vi "Demo_Main-User.vi"() -> ()   [LabVIEW 2010]
uses:
  ControlCAN/ControlCAN.llb/DevType.ctl
  ControlCAN/ControlCAN.llb/CAN Channel.ctl
  ControlCAN/ControlCAN.llb/InitFlag.ctl
  ControlCAN/ControlCAN.llb/Mode.ctl
  ControlCAN/ControlCAN.llb/Fliter.ctl
  ControlCAN/ControlCAN.llb/VCI_CAN_OBJ.ctl
  ControlCAN/ControlCAN.llb/VCI_INIT_CONFIG.ctl
  ControlCAN/ControlCAN.llb/Return Val.ctl
  ControlCAN/ControlCAN.lvlib
panel:
  out "版本号":dbl format="%_3f"
  in  "看门狗周期_R":bool
  in  "看门狗周期":u16
  out "看门狗周期_回":u16
  in  "看门狗周期_W":bool
  in  "看门狗_W":bool
  in  "看门狗":string(combo)="开启"
  in  "监测周期_R":bool
  in  "监测周期":u16
  out "监测周期_回":u16
  in  "监测周期_W":bool
  out "ERRO7":bool
  out "ERRO6":bool
  out "ERRO5":bool
  out "ERRO4":bool
  out "ERRO3":bool
  out "高温":bool
  out "高压":bool
  out "低压":bool
  out "warn7":bool
  out "warn6":bool
  out "warn5":bool
  out "warn4":bool
  out "warn3":bool
  out "高温":bool
  out "warn1":bool
  out "warn0":bool
  out "温度":dbl format="%#.6f"
  out "电机转速":dbl(graph)
  out "CAN ID":u8 format="%x"
  out "数组":u8[](array[numeric]) format="%x"
  in  "DATA_SAVE_W":bool
  out "CI_K0_回":u16
  out "BI_K0_回":u16
  in  "CI_K0_R":bool
  in  "BI_K0_R":bool
  in  "CI_K0_W":bool
  in  "BI_K0_W":bool
  in  "C电流零偏":u16
  in  "B电流零偏":u16
  in  "AI_K0_R":bool
  in  "A电流零偏":u16
  out "AI_K0_回":u16
  in  "AI_K0_W":bool
  out "Sin":i32
  out "Cosin":i32
  in  "加速度_R":bool
  in  "加速度":dbl min=0.0 max=8000.0 format="%#.6f"
  out "加速度_回":dbl format="%#.6f"
  in  "加速度_W":bool
  in  "速度环KI_R":bool
  in  "速度环KP_R":bool
  in  "速度环KI":dbl format="%#.6f"
  out "速度环KI_回":dbl format="%#.6f"
  in  "速度环KI_W":bool
  in  "速度环KP":dbl format="%#.6f"
  out "速度环KP_回":dbl format="%#.6f"
  in  "速度环KP_W":bool
  in  "电流环KI_R":bool
  in  "电流环KP_R":bool
  in  "电流环KI":dbl format="%#.6f"
  out "电流环KI_回":dbl format="%#.6f"
  in  "电流环KI_W":bool
  in  "电流环KP":dbl format="%#.6f"
  out "电流环KP_回":dbl format="%#.6f"
  in  "电流环KP_W":bool
  out "C电流":dbl(graph)
  out "B电流":dbl(graph)
  out "A电流":dbl(graph)
  out "sCnt":u32 caption="处理统计"
  out "模式_回":string(combo)="00"
  in  "模式_R":bool
  in  "设定电流_R":bool
  in  "设定位置_R":bool
  in  "设定速度_R":bool
  in  "存储路径":path
  in  "保存":bool
  out "保存_S":bool
  in  "模式_W":bool
  in  "模式":string(combo)="00"
  in  "设定电流":dbl format="%#.6f"
  out "设定电流_回":dbl format="%#.6f"
  in  "设定电流_W":bool
  in  "设定位置":dbl format="%#.6f"
  out "设定位置_回":dbl format="%#.6f"
  in  "设定位置_W":bool
  in  "设定速度":dbl format="%#.1f"
  out "设定速度_回":dbl format="%#.6f"
  in  "设定速度_W":bool
  in  "监测_W":bool
  in  "监测":string(combo)="30"
  out "电机ID_R":u32
  in  "Clear":bool
  out "Ualfa":dbl format="%#.6f"
  out "Ubate":dbl format="%#.6f"
  out "Uq":dbl format="%#.6f"
  out "Ud":dbl format="%#.6f"
  out "PWM1":u16
  out "PWM2":u16
  out "PWM3":u16
  out "sector":u8
  out "Iqnow":dbl
  out "Idnow":dbl
  out "Ialfa":dbl
  out "Ibeta":dbl
  out "A电流":dbl
  out "C电流":dbl
  out "B电流":dbl
  out "供电电压":dbl
  out "机械角度":dbl format="%.2f"
  out "电气角度":dbl
  out "转速":dbl
  out "CAN STD_ID":u32 format="%x"
  in  "电机ID":string(combo)="00"
  in  "电机ID_W":bool
  out "RecvCnt":u32 caption="接收统计"
  out "SendCnt":u32 caption="发送统计"
  in  "Format":u8(ring) items=["标准帧", "扩展帧"]
  in  "Type":u8(ring) items=["数据帧", "远程帧"]
  in  "Data":string="00 01 02 03 04 05 06 07"
  in  "ID":u32=291 format="0x%x"
  in  "Send":bool
  in  "RcvEnable":bool=TRUE
  out "Open":bool
  in  "Fliter":T1=1 items=["接收所有类型"=1, "只接收标准帧"=2, "只接收扩展帧"=3]
  in  "kBaudRate":u8(ring)=12 caption="波特率" items=["5k bps"=1, "10k bps"=2, "20k bps"=3, "40k bps"=4, "50k bps"=5, "80k bps"=6, "100k bps"=7, "125k bps"=8, "200k bps"=9, "250k bps"=10, "400k bps"=11, "500k bps"=12, "666k bps"=13, "800k bps"=14, "1000k bps"=15, "33.33k bps"=16, "66.66k bps"=17, "83.33k bps"=18]
  in  "Mode":T2 caption="工作模式" items=["正常工作", "仅侦听模式", "自测模式（环回）"]
  in  "InitFlag":T3 caption="初始化参数" items=["使用Flash参数", "使用界面设置参数"]
  in  "AccMask":u32=4294967295 caption="接收屏蔽码" format="%08x"
  in  "AccCode":u32 caption="接收过滤码" format="%08x"
  in  "Close":bool
  in  "Open":bool
  in  "Channel":T4 caption="CAN通道" items=["通道1", "通道2"]
  in  "DevType":T5=3 caption="设备类型" items=["USB-CAN"=2, "USB-CAN2"=3]
  # "CAN分析仪(创-芯-科-技)"
  # "CANalyst-II"
  # "发送指令帧包"
  # "CAN\n  ID"
  # "DATA"
  # "DATA"
  # "DATA"
  # "0"
  # "1"
  # "7"
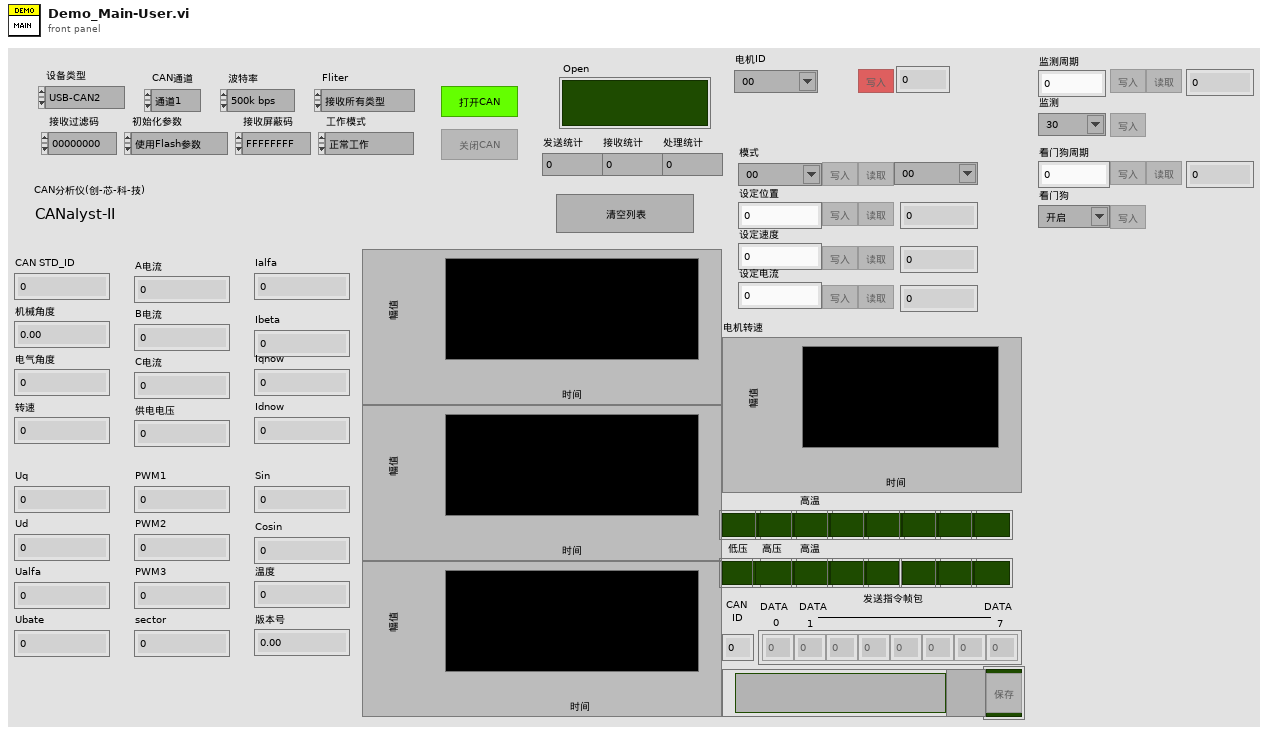
[diagram p1: front panel]
types:
  T1 = typedef "ControlCAN.lvlib/Fliter.ctl" = u8
  T2 = typedef "ControlCAN.lvlib/Mode.ctl" = u8
  T3 = typedef "ControlCAN.lvlib/InitFlag.ctl" = u32
  T4 = typedef "ControlCAN.lvlib/CAN Channel.ctl" = u32
  T5 = typedef "ControlCAN.lvlib/DevType.ctl" = u32
  T6 = typedef "ControlCAN.lvlib/VCI_CAN_OBJ.ctl" = cluster{"ID":u32, "TimeStamp":u32, "TimeFlag":u8, "SendType":u8, "RemoteFlag":u8, "ExternFlag":u8, "DataLen":u8, "Data":u8[], "Reserved":u8[]}
  T7 = cluster{"Type":enum16{"接收", "发送"}, "Channel":T4, "Time":timestamp, "VCI_CAN_OBJ":T6}[]
  T8 = typedef "ControlCAN.lvlib/VCI_INIT_CONFIG.ctl" = cluster{"AccCode":u32, "AccMask":u32, "InitFlag":T3, "Fliter":T1, "Timing0":u8, "Timing1":u8, "Mode":T2}
  T9 = cluster{"DevType":T5, "DevIndex":u32, "CanIndex":T4, "VCI_INIT_CONFIG":T8}
  T10 = typedef "ControlCAN.lvlib/Return Val.ctl" = i32
  T11 = enum16{"open", "replace", "create", "open or create", "replace or create", "replace or create with confirmation"}
  T12 = cluster{"[0]":cluster{"Type":enum16{"接收", "发送"}, "Channel":T4, "Time":timestamp, "VCI_CAN_OBJ":T6}}
  T13 = cluster{"Type":enum16{"接收", "发送"}, "Channel":T4, "Time":timestamp, "VCI_CAN_OBJ":T6}
  T14 = cluster{"Data[0]":u8, "Data[1]":u8, "Data[2]":u8, "Data[3]":u8, "Data[4]":u8, "Data[5]":u8, "Data[6]":u8, "Data[7]":u8}
  T15 = cluster{"Boolean array[0]":bool, "Boolean array[1]":bool, "Boolean array[2]":bool, "Boolean array[3]":bool, "Boolean array[4]":bool, "Boolean array[5]":bool, "Boolean array[6]":bool, "Boolean array[7]":bool}
  T16 = enum32{"invalid app kind", "Development System", "Run Time System", "Student Edition", "Embedded LabVIEW", "Evaluation", "Custom"}
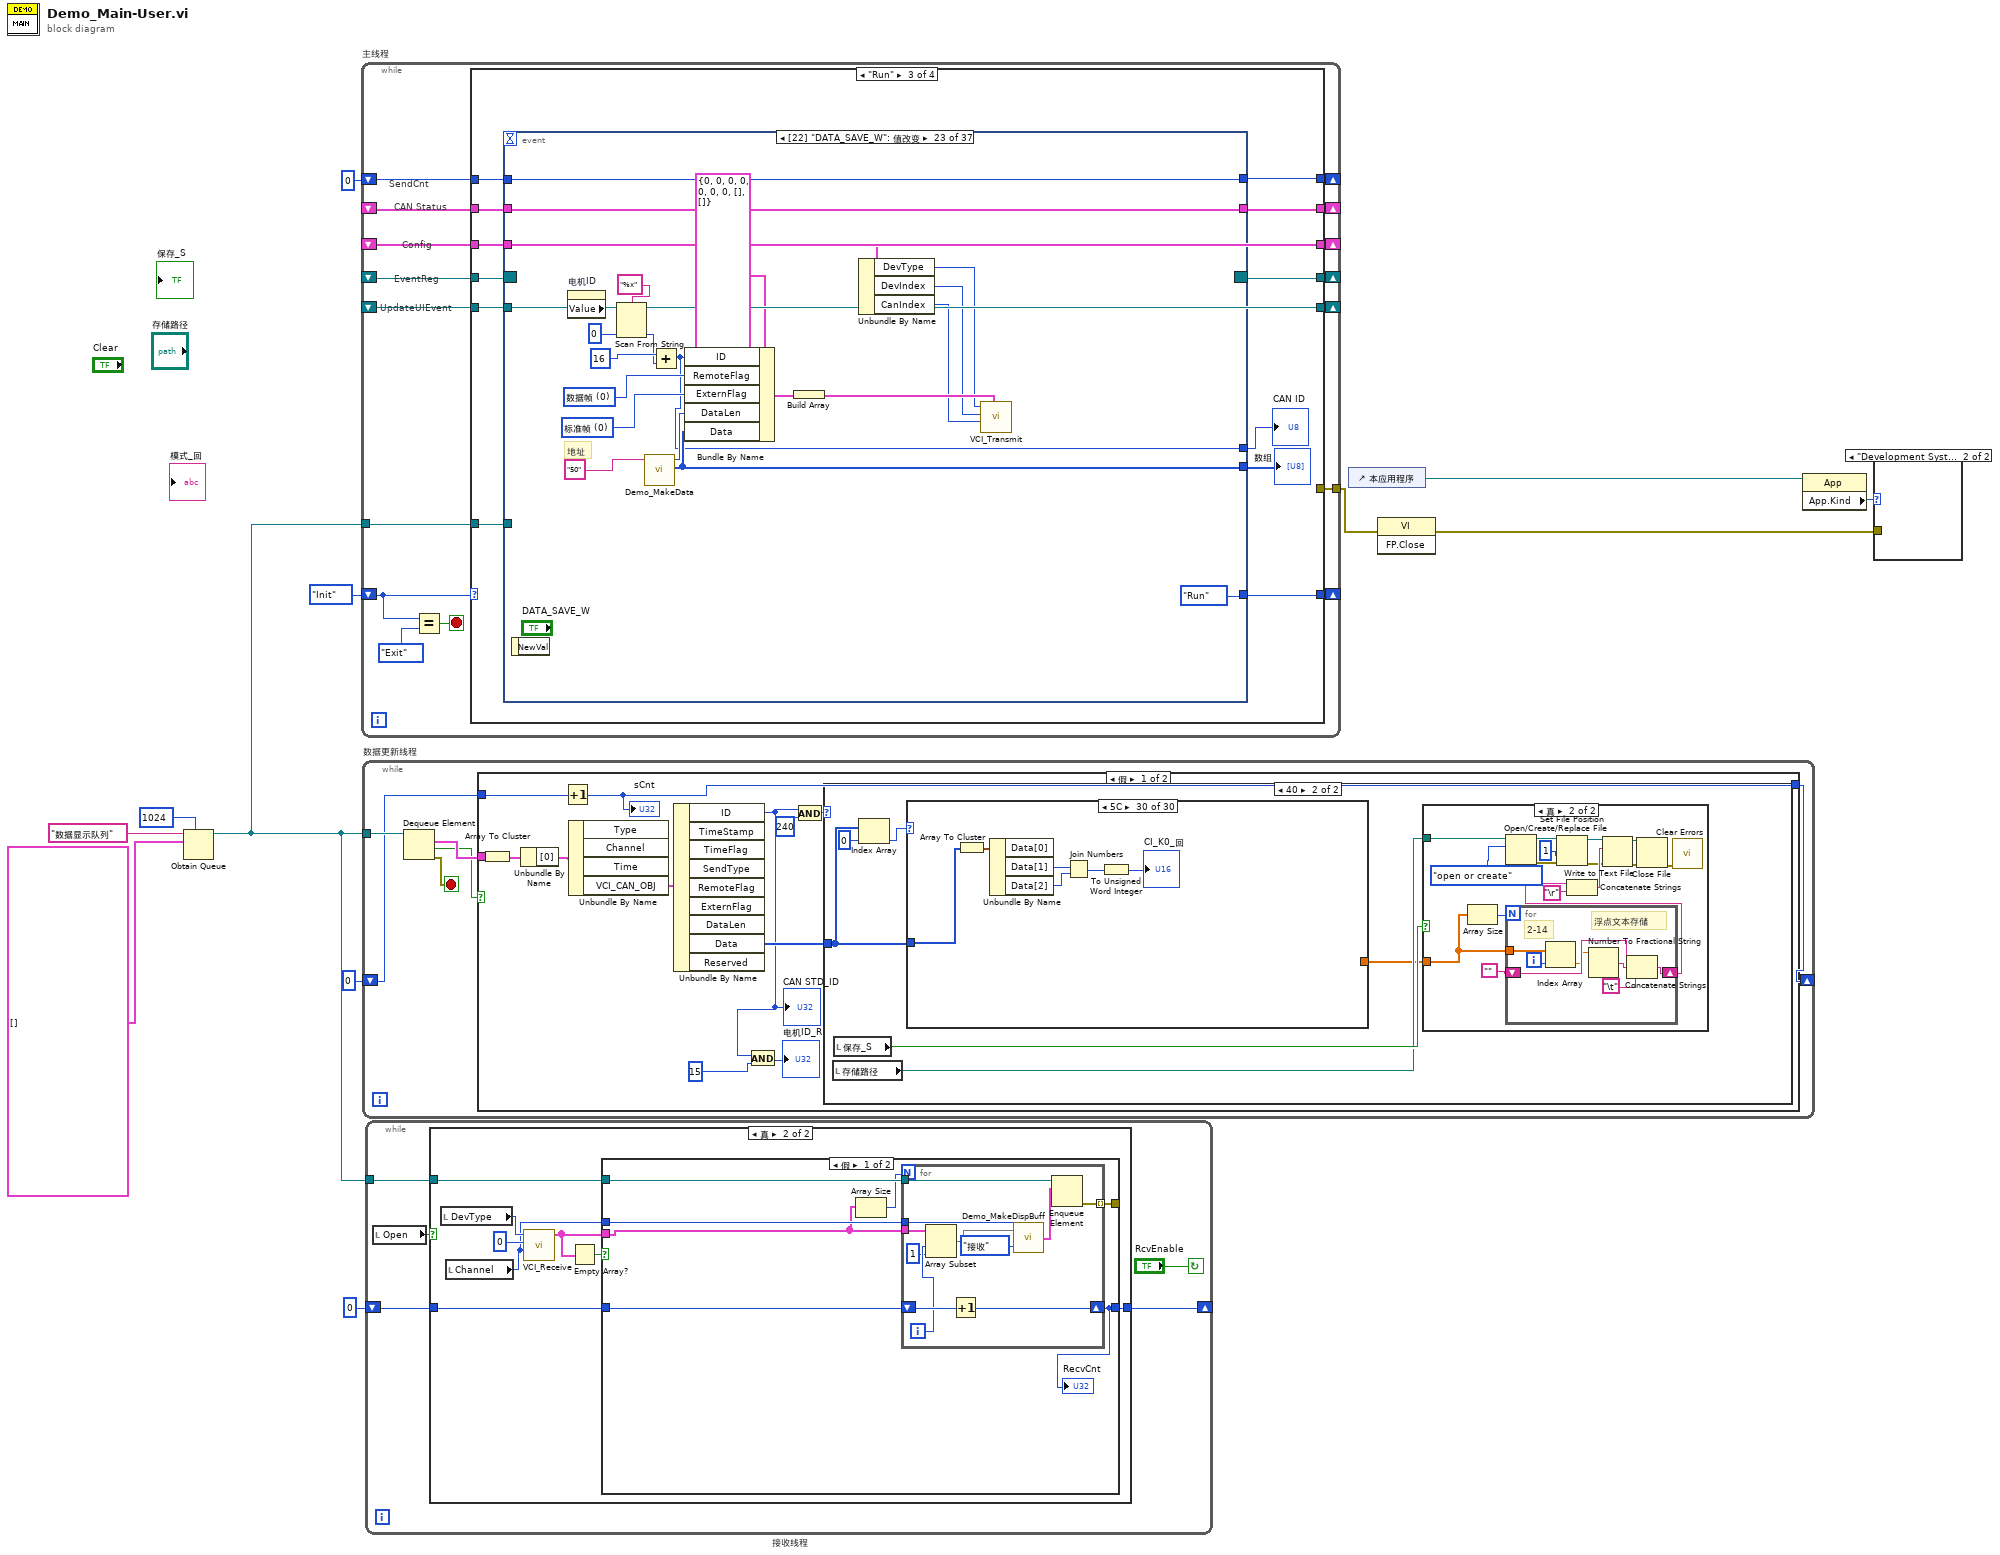
[diagram p0: block diagram]
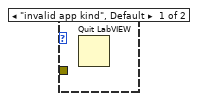
[diagram p2: hidden frame]
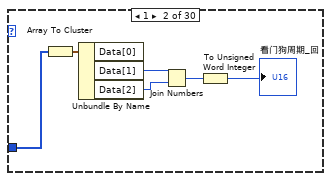
[diagram p6: hidden frame]
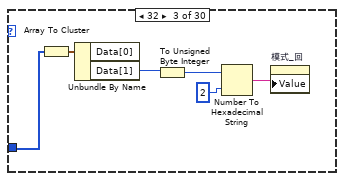
[diagram p7: hidden frame]
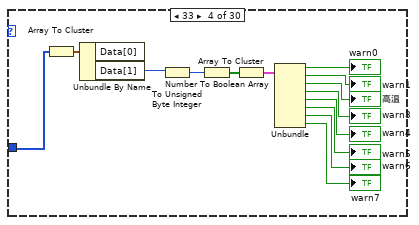
[diagram p8: hidden frame]
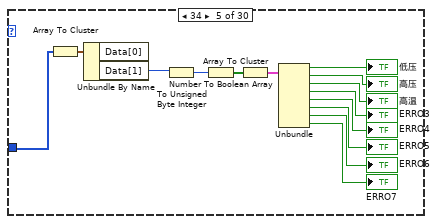
[diagram p9: hidden frame]
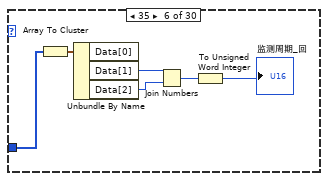
[diagram p10: hidden frame]
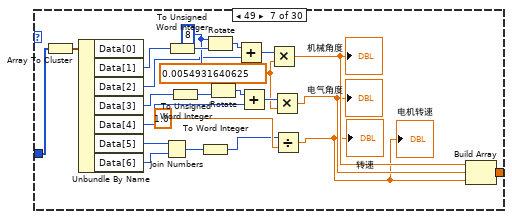
[diagram p11: hidden frame]
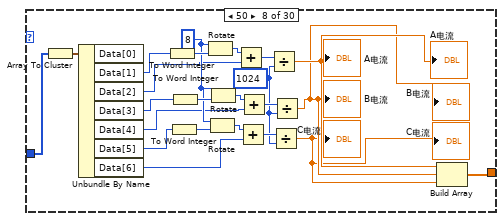
[diagram p12: hidden frame]
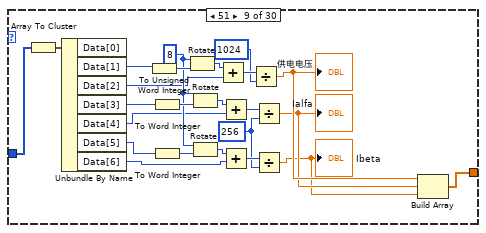
[diagram p13: hidden frame]
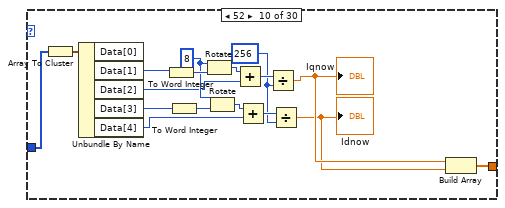
[diagram p14: hidden frame]
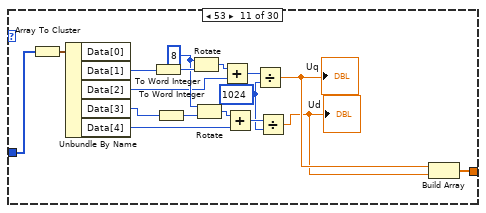
[diagram p15: hidden frame]
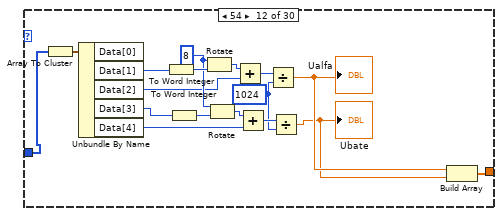
[diagram p16: hidden frame]
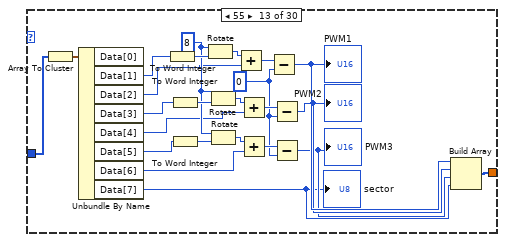
[diagram p17: hidden frame]
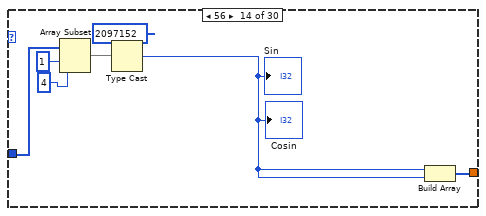
[diagram p18: hidden frame]
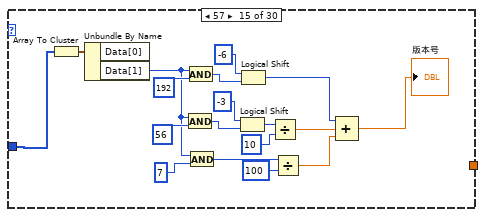
[diagram p19: hidden frame]
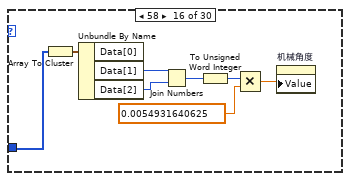
[diagram p20: hidden frame]
diagram:
  n1 = Obtain Queue(max queue size (-1, unlimited)=1024, name (unnamed)="数据显示队列" ("名称（未命名）"), element data type=T7 []) -> (queue out=w9:refnum<queue>)  [unwired: 2 in, 2 out]
  n2 = while "主线程" {
    shift-right: [w24] -> _
    shift-left: enum16{"Init", "Wait", "Run", "Exit"}."Init" -> [w27]
    shift-right: [w25] -> _
    shift-left: _ -> [w26]
    shift-right: [w23] -> _
    shift-left: _ -> [w22]
    tunnel: w9 -> [w21]
    shift-right: [w19] -> _
    shift-left: _ -> [w18]
    shift-right: [w17] -> _
    shift-left: _ -> [w16]
    shift-right: [w14] -> _
    shift-left: u32 0 -> [w15]
    tunnel: [w13] -> w4
    stop <- w28 stop-if-true
    # "CAN Status"
    # "Config"
    # "EventReg"
    # "UpdateUIEvent"
    # "SendCnt"
    n3 = Equal?(x=w27, y=enum16{"Init", "Wait", "Run", "Exit"}."Exit") -> (x = y?=w28:bool)
    n4 = case shown="\"Run\"" w27 {
      tunnel: w26 -> [_ w57 w158 w968]
      tunnel: [w48 w56 w157 w968] -> w25
      tunnel: [enum16{"Init", "Wait", "Run", "Exit"}."Wait" w53 w160 enum16{"Init", "Wait", "Run", "Exit"}."Exit"] -> w24
      tunnel: [w44 w54 w156 w966] -> w23
      tunnel: w22 -> [_ w55 w156 w966]
      tunnel: w21 -> [_ w52 w159 w972]
      tunnel: [w36 w51 w154 w971] -> w19
      tunnel: w18 -> [_ w51 w155 w971]
      tunnel: [w35 w50 w153 w969] -> w17
      tunnel: w16 -> [_ w50 w153 w969]
      tunnel: w15 -> [w33 w49 w152 w964]
      tunnel: [w33 w49 w151 w964] -> w14
      tunnel: [_ _ _ errorcluster {"status"=FALSE, "code"=0, "source"=""} ("error constant")] -> w13
      frame "Init", Default {
        w37 = cluster{"CANOpen":bool} {"CANOpen"=FALSE}  # UpdateUI
        w47 = T9 {"DevType"=2, "DevIndex"=0, "CanIndex"=0, "VCI_INIT_CONFIG"={"AccCode"=0, "AccMask"=0, "InitFlag"=0, "Fliter"=0, "Timing0"=0, "Timing1"=0, "Mode"=0}}  # Config
        w48 = cluster{"Open":bool, "SendCnt":u32} {"Open"=FALSE, "SendCnt"=0}  # CAN Status
        n5 = property class="VI"("Front Panel.Closeable"=TRUE ("前面板窗口:可关闭")) -> ()  [unwired: 2 in, 2 out]
        n6 = invoke class="VI" method="Default Vals.Reinit All"() -> ()  [unwired: 3 in, 3 out]
        n7 = call "Demo_GetT0T1.vi"("kBaudRate"="kBaudRate") -> ("Timing0"=w30:u8, "Timing1"=w29:u8)
        n8 = Bundle By Name(cluster=w47, "DevType"="DevType", "CanIndex"="Channel", "VCI_INIT_CONFIG.AccCode"="AccCode", "VCI_INIT_CONFIG.AccMask"="AccMask", "VCI_INIT_CONFIG.InitFlag"="InitFlag", "VCI_INIT_CONFIG.Fliter"="Fliter", "VCI_INIT_CONFIG.Timing0"=w30, "VCI_INIT_CONFIG.Timing1"=w29, "VCI_INIT_CONFIG.Mode"="Mode") -> (w44:T9)
        n9 = local write "RcvEnable"(TRUE ("RcvEnable")) -> ()
        n10 = Create User Event(user event datatype=w37) -> (user event=w35:refnum<user-event>)  [unwired: 1 in, 1 out]
        n11 = register-events(w35) -> (reference out=w36:refnum<event-registration>)  [unwired: 2 in, 1 out]
      }
      frame "Wait" {
        n12 = event shown="[1] 前面板关闭？" {
          selector: _ -> [_ _ _ _ _ _ _ _ _ _]
          dyn-events: _ -> [_ _ _ _ _ _ _ _ _ _]
          timeout: _ -> [_ _ _ _ _ _ _ _ _ _]
          tunnel: w57 -> [w61 w101 w111 w116 w121 w126 w131 w136 w143 w148]
          tunnel: [w60 w101 w111 w116 w121 w126 w131 w136 w143 w148] -> w56
          tunnel: w55 -> [w71 w100 w110 w115 w120 w125 w130 w135 w142 w147]
          tunnel: [w71 w100 w109 w113 w118 w123 w128 w133 w141 w145] -> w54
          tunnel: [w62 enum16{"Init", "Wait", "Run", "Exit"}."Exit" enum16{"Init", "Wait", "Run", "Exit"}."Wait" enum16{"Init", "Wait", "Run", "Exit"}."Wait" enum16{"Init", "Wait", "Run", "Exit"}."Wait" enum16{"Init", "Wait", "Run", "Exit"}."Wait" enum16{"Init", "Wait", "Run", "Exit"}."Wait" enum16{"Init", "Wait", "Run", "Exit"}."Wait" enum16{"Init", "Wait", "Run", "Exit"}."Wait" enum16{"Init", "Wait", "Run", "Exit"}."Wait"] -> w53
          tunnel: w52 -> [_ _ _ _ _ _ _ _ _ _]
          tunnel: w50 -> [w59 _ _ _ _ _ _ _ _ _]
          event "Open": Value Change {
            w65 = T10 1 items=["OK"=1, "ERROR1"=0, "ERROR2"=-1] ("y")
            # "打开CAN的步骤：\n1.Open\n2.Init\n3.Start"
            n13 = event-data() -> ()  [unwired: 2 out]
            n14 = Unbundle By Name(w71) -> ("DevType"=w70:T5, "DevIndex"=w69:u32)
            n15 = call "VCI_OpenDevice.vi"("DevIndex"=w69, "DevType"=w70) -> ("error out"=w66:errorcluster, "Return Val"=w68:T10)  [unwired: 2 in, 6 out]
            n16 = Equal?(x=w68, y=w65) -> (x = y?=w67:bool)
            n17 = case shown="真" w67 {
              tunnel: w66 -> [_ w86]
              tunnel: w71 -> [_ w85]
              tunnel: w65 -> [_ w77]
              tunnel: [_ w76] -> w58
              frame False {
              }
              frame True {
                n18 = Unbundle By Name(w85) -> ("VCI_INIT_CONFIG"=w84:T8, "DevType"=w80:T5, "DevIndex"=w79:u32, "CanIndex"=w78:T4)
                n19 = call "VCI_InitCAN.vi"("VCI_INIT_CONFIG"=w84, "error in (no error)"=w86, "CANIndex"=w78, "DevIndex"=w79, "DevType"=w80) -> ("error out"=w81:errorcluster, "Return Val"=w83:T10)  [unwired: 5 out]
                n20 = Equal?(x=w77, y=w83) -> (x = y?=w82:bool)
                n21 = case shown="真" w82 {
                  tunnel: w81 -> [_ w97]
                  tunnel: w80 -> [_ w96]
                  tunnel: w79 -> [_ w95]
                  tunnel: w78 -> [_ w94]
                  tunnel: w77 -> [_ w92]
                  tunnel: [_ w88] -> w76
                  frame False {
                  }
                  frame True {
                    n22 = call "VCI_StartCAN.vi"("error in (no error)"=w97, "CANIndex"=w94, "DevIndex"=w95, "DevType"=w96) -> ("error out"=w90:errorcluster, "Return Val"=w93:T10)  [unwired: 6 out]
                    n23 = Unbundle By Name(w90) -> ("status"=w87:bool)
                    n24 = Equal?(x=w92, y=w93) -> (x = y?=w91:bool)
                    n25 = Not(x=w87) -> (.not. x?=w89:bool)
                    n26 = And(x=w91, y=w89) -> (x .and. y?=w88:bool)
                  }
                }
              }
            }
            n27 = case shown="真" w58 {
              tunnel: w59 -> [_ w75]
              tunnel: w58 -> [_ w73]
              frame False {
              }
              frame True {
                n28 = Bundle By Name(cluster=cluster{"CANOpen":bool} {"CANOpen"=FALSE} ("事件数据"), "CANOpen"=w73) -> (w72:cluster{"CANOpen":bool})
                n29 = Generate User Event(user event=w75, event data cluster=w72) -> ()  [unwired: 1 in, 2 out]
              }
            }
            n30 = Select(t=enum16{"Init", "Wait", "Run", "Exit"}."Run", s=w58, f=enum16{"Init", "Wait", "Run", "Exit"}."Wait") -> (s? t:f=w62:enum16{"Init", "Wait", "Run", "Exit"})
            n31 = Bundle By Name(cluster=w61, "Open"=w58) -> (w60:cluster{"Open":bool, "SendCnt":u32})
          }
          event Panel Close? {
            n32 = event-data() -> ()  [unwired: 2 out]
            n33 = event-data("Discard?"=TRUE ("放弃？")) -> ()  [unwired: 1 in, 1 out]
          }
          event Value Change {
            w107 = T5 3 items=["USB-CAN"=2, "USB-CAN2"=3] ("y")
            n34 = event-data() -> ("NewVal"=w108:T5)  [unwired: 1 out]
            n35 = Equal?(x=w108, y=w107) -> (x = y?=w106:bool)
            n36 = Bundle By Name(cluster=w110, "DevType"=w108) -> (w109:T9)
            n37 = Select(t=i32[] [] ("禁用项[]"), s=w106, f=i32[] [1] ("禁用项[]")) -> (s? t:f=w105:i32[])
            n38 = property on="Channel" class="Ring (严格)"("Disabled Items []"=w105) -> ()  [unwired: 2 in, 2 out]
          }
          event Value Change {
            n39 = event-data() -> ("NewVal"=w114:T4)  [unwired: 1 out]
            n40 = Bundle By Name(cluster=w115, "CanIndex"=w114) -> (w113:T9)
          }
          event "AccCode": Value Change {
            n41 = event-data() -> ("NewVal"=w119:u32)  [unwired: 1 out]
            n42 = Bundle By Name(cluster=w120, "VCI_INIT_CONFIG.AccCode"=w119) -> (w118:T9)
          }
          event "AccMask": Value Change {
            n43 = event-data() -> ("NewVal"=w124:u32)  [unwired: 1 out]
            n44 = Bundle By Name(cluster=w125, "VCI_INIT_CONFIG.AccMask"=w124) -> (w123:T9)
          }
          event Value Change {
            n45 = event-data() -> ("NewVal"=w129:T3)  [unwired: 1 out]
            n46 = Bundle By Name(cluster=w130, "VCI_INIT_CONFIG.InitFlag"=w129) -> (w128:T9)
          }
          event Value Change {
            n47 = event-data() -> ("NewVal"=w134:T2)  [unwired: 1 out]
            n48 = Bundle By Name(cluster=w135, "VCI_INIT_CONFIG.Mode"=w134) -> (w133:T9)
          }
          event "kBaudRate": Value Change {
            n49 = event-data() -> ("NewVal"=w139:u8)  [unwired: 1 out]
            n50 = call "Demo_GetT0T1.vi"("kBaudRate"=w139) -> ("Timing0"=w138:u8, "Timing1"=w137:u8)
            n51 = Bundle By Name(cluster=w142, "VCI_INIT_CONFIG.Timing0"=w138, "VCI_INIT_CONFIG.Timing1"=w137) -> (w141:T9)
          }
          event Value Change {
            n52 = event-data() -> ("NewVal"=w146:T1)  [unwired: 1 out]
            n53 = Bundle By Name(cluster=w147, "VCI_INIT_CONFIG.Fliter"=w146) -> (w145:T9)
          }
        }
      }
      frame "Run" {
        n54 = event shown="[22] \"DATA_SAVE_W\": 值改变" {
          selector: w155 -> [_ _ _ _ _ _ _ _ _ _ _ _ _ _ _ _ _ _ _ _ _ _ _ _ _ _ _ _ _ _ _ _ _ _ _ _ _]
          dyn-events: [_ _ _ _ _ _ _ _ _ _ _ _ _ _ _ _ _ _ _ _ _ _ _ _ _ _ _ _ _ _ _ _ _ _ _ _ _] -> w154
          timeout: _ -> [_ _ _ _ _ _ _ _ _ _ _ _ _ _ _ _ _ _ _ _ _ _ _ _ _ _ _ _ _ _ _ _ _ _ _ _ _]
          tunnel: [enum16{"Init", "Wait", "Run", "Exit"}."Run" enum16{"Init", "Wait", "Run", "Exit"}."Run" enum16{"Init", "Wait", "Run", "Exit"}."Run" enum16{"Init", "Wait", "Run", "Exit"}."Run" enum16{"Init", "Wait", "Run", "Exit"}."Run" enum16{"Init", "Wait", "Run", "Exit"}."Run" enum16{"Init", "Wait", "Run", "Exit"}."Run" enum16{"Init", "Wait", "Run", "Exit"}."Run" enum16{"Init", "Wait", "Run", "Exit"}."Run" enum16{"Init", "Wait", "Run", "Exit"}."Run" enum16{"Init", "Wait", "Run", "Exit"}."Run" enum16{"Init", "Wait", "Run", "Exit"}."Run" enum16{"Init", "Wait", "Run", "Exit"}."Run" enum16{"Init", "Wait", "Run", "Exit"}."Run" enum16{"Init", "Wait", "Run", "Exit"}."Run" enum16{"Init", "Wait", "Run", "Exit"}."Run" enum16{"Init", "Wait", "Run", "Exit"}."Run" enum16{"Init", "Wait", "Run", "Exit"}."Run" enum16{"Init", "Wait", "Run", "Exit"}."Run" enum16{"Init", "Wait", "Run", "Exit"}."Run" enum16{"Init", "Wait", "Run", "Exit"}."Run" enum16{"Init", "Wait", "Run", "Exit"}."Run" enum16{"Init", "Wait", "Run", "Exit"}."Run" enum16{"Init", "Wait", "Run", "Exit"}."Run" enum16{"Init", "Wait", "Run", "Exit"}."Run" enum16{"Init", "Wait", "Run", "Exit"}."Run" enum16{"Init", "Wait", "Run", "Exit"}."Run" enum16{"Init", "Wait", "Run", "Exit"}."Run" enum16{"Init", "Wait", "Run", "Exit"}."Run" enum16{"Init", "Wait", "Run", "Exit"}."Run" enum16{"Init", "Wait", "Run", "Exit"}."Run" enum16{"Init", "Wait", "Run", "Exit"}."Run" enum16{"Init", "Wait", "Run", "Exit"}."Run" enum16{"Init", "Wait", "Run", "Exit"}."Run" enum16{"Init", "Wait", "Run", "Exit"}."Run" enum16{"Init", "Wait", "Run", "Exit"}."Run" w957] -> w160
          tunnel: w159 -> [_ _ _ _ _ _ _ _ _ _ _ _ _ _ _ _ _ _ _ _ _ _ _ _ _ _ _ _ _ _ _ _ _ _ _ _ _]
          tunnel: [w162 w179 w196 w220 w241 w262 w281 w302 w318 w356 w377 w403 w429 w455 w481 w507 w533 w559 w585 w609 w633 w657 w678 w699 w720 w741 w762 w783 w804 w825 w846 w867 w888 w909 w937 w943 w962] -> w157
          tunnel: w158 -> [w162 w179 w196 w220 w241 w262 w281 w302 w318 w356 w377 w403 w429 w455 w481 w507 w533 w559 w585 w609 w633 w657 w678 w699 w720 w741 w762 w783 w804 w825 w846 w867 w888 w909 w937 w945 w962]
          tunnel: w156 -> [_ w174 w186 w201 w224 w251 w267 w285 w308 w338 w360 w388 w411 w437 w460 w486 w512 w538 w564 w590 w614 w638 w661 w682 w703 w724 w745 w766 w787 w808 w829 w850 w871 w892 _ w950 _]
          tunnel: w153 -> [_ _ _ _ _ _ _ _ _ _ _ _ _ _ _ _ _ _ _ _ _ _ _ _ _ _ _ _ _ _ _ _ _ _ _ w942 _]
          tunnel: w152 -> [w161 w167 w195 w219 w240 w261 w280 w301 w317 w355 w376 w402 w428 w454 w480 w506 w532 w558 w584 w608 w632 w656 w677 w698 w719 w740 w761 w782 w803 w824 w845 w866 w887 w908 w936 w938 w956]
          tunnel: [w161 w166 w195 w219 w240 w261 w280 w301 w317 w355 w376 w402 w428 w454 w480 w506 w532 w558 w584 w608 w632 w656 w677 w698 w719 w740 w761 w782 w803 w824 w845 w866 w887 w908 w936 w938 w956] -> w151
          tunnel: [_ _ w182 w199 w222 w243 w265 w283 w304 w336 w358 w379 w405 w431 w457 w483 w509 w535 w561 w587 w611 w635 w659 w680 w701 w722 w743 w764 w785 w806 w827 w848 w869 w890 _ _ _] -> w150
          tunnel: [_ _ w181 w200 w223 w242 w266 w284 w307 w335 w357 w378 w404 w430 w456 w482 w508 w534 w560 w586 w610 w634 w658 w679 w700 w721 w742 w763 w784 w805 w826 w847 w868 w889 _ _ _] -> w149
          event Timeout {
            n55 = event-data() -> ()  [unwired: 3 out]
          }
          event "Send": Value Change {
            n56 = event-data() -> ()  [unwired: 2 out]
            n57 = Increment(x=w167) -> (x+1=w166:u32)
            "SendCnt" <- w166
            n58 = call "Demo_MakeData.vi"("DataString"="Data") -> ("Data"=w169:u8[], "DataLen"=w170:u8)  [unwired: 9 out]
            n59 = Bundle By Name(cluster=T6 {"ID"=0, "TimeStamp"=0, "TimeFlag"=0, "SendType"=0, "RemoteFlag"=0, "ExternFlag"=0, "DataLen"=0, "Data"=[], "Reserved"=[]} ("Send"), "ID"="ID", "RemoteFlag"="Type", "ExternFlag"="Format", "DataLen"=w170, "Data"=w169) -> (w164:T6)
            n60 = Build Array(w164) -> (w165:T6[])
            n61 = Unbundle By Name(w174) -> ("DevType"=w173:T5, "DevIndex"=w172:u32, "CanIndex"=w168:T4)
            n62 = call "VCI_Transmit.vi"("Buffer"=w165, "CANIndex"=w168, "DevIndex"=w172, "DevType"=w173) -> ()  [unwired: 1 in, 7 out]
          }
          event "电机ID_W": Value Change {
            w185 = u8 0 items=["数据帧", "遥控帧"]
            w181 = u32 138
            w184 = u8 0 items=["标准帧", "扩展帧"]
            n63 = event-data() -> ()  [unwired: 2 out]
            n64 = call "Demo_MakeData.vi"("DataString"="电机ID") -> ("Data"=w182:u8[], "DataLen"=w190:u8)  [unwired: 9 out]
            n65 = Bundle By Name(cluster=T6 {"ID"=0, "TimeStamp"=0, "TimeFlag"=0, "SendType"=0, "RemoteFlag"=0, "ExternFlag"=0, "DataLen"=0, "Data"=[], "Reserved"=[]} ("Send"), "ID"=w181, "RemoteFlag"=w185, "ExternFlag"=w184, "DataLen"=w190, "Data"=w182) -> (w187:T6)
            n66 = Build Array(w187) -> (w188:T6[])
            n67 = Unbundle By Name(w186) -> ("DevType"=w192:T5, "DevIndex"=w191:u32, "CanIndex"=w189:T4)
            n68 = call "VCI_Transmit.vi"("Buffer"=w188, "CANIndex"=w189, "DevIndex"=w191, "DevType"=w192) -> ()  [unwired: 1 in, 7 out]
          }
          event "监测周期_W": Value Change {
            w213 = u8 0 items=["数据帧", "遥控帧"]
            w214 = u8 0 items=["标准帧", "扩展帧"]
            # "索引地址"
            n69 = event-data() -> ()  [unwired: 2 out]
            n70 = property on="电机ID" class="CmbBox"() -> ("Value"=w205:string)  [unwired: 2 in, 2 out]
            n71 = Scan From String(format string="%x" ("格式字符串"), input string=w205, default 1=u8 0) -> (output 1=w202:u8)  [unwired: 2 in, 3 out]
            n72 = Split Number(x="监测周期") -> (hi(x)=w217:u8, lo(x)=w218:u8)
            n73 = Add(x=u32 16, y=w202) -> (x+y=w200:u32)
            n74 = Build Array(u8 35, w217, w218) -> (w199:u8[])
            n75 = Bundle By Name(cluster=T6 {"ID"=0, "TimeStamp"=0, "TimeFlag"=0, "SendType"=0, "RemoteFlag"=0, "ExternFlag"=0, "DataLen"=0, "Data"=[], "Reserved"=[]} ("Send"), "ID"=w200, "RemoteFlag"=w213, "ExternFlag"=w214, "DataLen"=u8 3, "Data"=w199) -> (w212:T6)
            n76 = Build Array(w212) -> (w211:T6[])
            n77 = Unbundle By Name(w201) -> ("DevType"=w208:T5, "DevIndex"=w209:u32, "CanIndex"=w210:T4)
            n78 = call "VCI_Transmit.vi"("Buffer"=w211, "CANIndex"=w210, "DevIndex"=w209, "DevType"=w208) -> ()  [unwired: 1 in, 7 out]
          }
          event "监测周期_R": Value Change {
            w237 = u8 0 items=["数据帧", "遥控帧"]
            w238 = u8 0 items=["标准帧", "扩展帧"]
            # "地址"
            n79 = event-data() -> ()  [unwired: 2 out]
            n80 = property on="电机ID" class="CmbBox"() -> ("Value"=w228:string)  [unwired: 2 in, 2 out]
            n81 = Scan From String(format string="%x" ("格式字符串"), input string=w228, default 1=u8 0) -> (output 1=w225:u8)  [unwired: 2 in, 3 out]
            n82 = call "Demo_MakeData.vi"("DataString"="23 ") -> ("Data"=w222:u8[], "DataLen"=w233:u8)  [unwired: 9 out]
            n83 = Add(x=u32 48, y=w225) -> (x+y=w223:u32)
            n84 = Bundle By Name(cluster=T6 {"ID"=0, "TimeStamp"=0, "TimeFlag"=0, "SendType"=0, "RemoteFlag"=0, "ExternFlag"=0, "DataLen"=0, "Data"=[], "Reserved"=[]} ("Send"), "ID"=w223, "RemoteFlag"=w237, "ExternFlag"=w238, "DataLen"=w233, "Data"=w222) -> (w236:T6)
            n85 = Build Array(w236) -> (w235:T6[])
            n86 = Unbundle By Name(w224) -> ("DevType"=w231:T5, "DevIndex"=w232:u32, "CanIndex"=w234:T4)
            n87 = call "VCI_Transmit.vi"("Buffer"=w235, "CANIndex"=w234, "DevIndex"=w232, "DevType"=w231) -> ()  [unwired: 1 in, 7 out]
          }
          event "监测_W": Value Change {
            w259 = u8 0 items=["数据帧", "遥控帧"]
            w260 = u8 0 items=["标准帧", "扩展帧"]
            # "地址"
            n88 = event-data() -> ()  [unwired: 2 out]
            n89 = property on="电机ID" class="CmbBox"() -> ("Value"=w248:string)  [unwired: 2 in, 2 out]
            n90 = Scan From String(format string="%x" ("格式字符串"), input string=w248, default 1=u8 0) -> (output 1=w245:u8)  [unwired: 2 in, 3 out]
            n91 = call "Demo_MakeData.vi"("DataString"="监测") -> ("Data"=w243:u8[], "DataLen"=w255:u8)  [unwired: 9 out]
            n92 = Add(x=u32 48, y=w245) -> (x+y=w242:u32)
            n93 = Bundle By Name(cluster=T6 {"ID"=0, "TimeStamp"=0, "TimeFlag"=0, "SendType"=0, "RemoteFlag"=0, "ExternFlag"=0, "DataLen"=0, "Data"=[], "Reserved"=[]} ("Send"), "ID"=w242, "RemoteFlag"=w259, "ExternFlag"=w260, "DataLen"=w255, "Data"=w243) -> (w258:T6)
            n94 = Build Array(w258) -> (w257:T6[])
            n95 = Unbundle By Name(w251) -> ("DevType"=w253:T5, "DevIndex"=w254:u32, "CanIndex"=w256:T4)
            n96 = call "VCI_Transmit.vi"("Buffer"=w257, "CANIndex"=w256, "DevIndex"=w254, "DevType"=w253) -> ()  [unwired: 1 in, 7 out]
          }
          event "看门狗周期_W": Value Change {
            w273 = u8 0 items=["数据帧", "遥控帧"]
            w272 = u8 0 items=["标准帧", "扩展帧"]
            w266 = u32 138
            # "索引地址"
            n97 = event-data() -> ()  [unwired: 2 out]
            n98 = Split Number(x="看门狗周期") -> (hi(x)=w269:u8, lo(x)=w268:u8)
            n99 = Build Array(u8 1, w269, w268) -> (w265:u8[])
            n100 = Bundle By Name(cluster=T6 {"ID"=0, "TimeStamp"=0, "TimeFlag"=0, "SendType"=0, "RemoteFlag"=0, "ExternFlag"=0, "DataLen"=0, "Data"=[], "Reserved"=[]} ("Send"), "ID"=w266, "RemoteFlag"=w273, "ExternFlag"=w272, "DataLen"=u8 3, "Data"=w265) -> (w274:T6)
            n101 = Build Array(w274) -> (w275:T6[])
            n102 = Unbundle By Name(w267) -> ("DevType"=w278:T5, "DevIndex"=w277:u32, "CanIndex"=w276:T4)
            n103 = call "VCI_Transmit.vi"("Buffer"=w275, "CANIndex"=w276, "DevIndex"=w277, "DevType"=w278) -> ()  [unwired: 1 in, 7 out]
          }
          event "看门狗周期_R": Value Change {
            w288 = u8 0 items=["数据帧", "遥控帧"]
            w287 = u8 0 items=["标准帧", "扩展帧"]
            # "地址"
            n104 = event-data() -> ()  [unwired: 2 out]
            n105 = property on="电机ID" class="CmbBox"() -> ("Value"=w297:string)  [unwired: 2 in, 2 out]
            n106 = Scan From String(format string="%x" ("格式字符串"), input string=w297, default 1=u8 0) -> (output 1=w300:u8)  [unwired: 2 in, 3 out]
            n107 = call "Demo_MakeData.vi"("DataString"="01") -> ("Data"=w283:u8[], "DataLen"=w292:u8)  [unwired: 9 out]
            n108 = Add(x=u32 48, y=w300) -> (x+y=w284:u32)
            n109 = Bundle By Name(cluster=T6 {"ID"=0, "TimeStamp"=0, "TimeFlag"=0, "SendType"=0, "RemoteFlag"=0, "ExternFlag"=0, "DataLen"=0, "Data"=[], "Reserved"=[]} ("Send"), "ID"=w284, "RemoteFlag"=w288, "ExternFlag"=w287, "DataLen"=w292, "Data"=w283) -> (w289:T6)
            n110 = Build Array(w289) -> (w290:T6[])
            n111 = Unbundle By Name(w285) -> ("DevType"=w294:T5, "DevIndex"=w293:u32, "CanIndex"=w291:T4)
            n112 = call "VCI_Transmit.vi"("Buffer"=w290, "CANIndex"=w291, "DevIndex"=w293, "DevType"=w294) -> ()  [unwired: 1 in, 7 out]
          }
          event "看门狗_W": Value Change {
            w315 = u8 0 items=["数据帧", "遥控帧"]
            w307 = u32 138
            w316 = u8 0 items=["标准帧", "扩展帧"]
            n113 = event-data() -> ()  [unwired: 2 out]
            n114 = case shown="\"开启\", 默认" "看门狗" {
              tunnel: [w319 w324 w329] -> w304
              frame "开启", Default {
                n115 = Split Number(x=u16 52428) -> (hi(x)=w322:u8, lo(x)=w323:u8)
                n116 = Build Array(u8 2, w322, w323) -> (w319:u8[])
              }
              frame "喂狗" {
                n117 = Split Number(x=u16 43690) -> (hi(x)=w326:u8, lo(x)=w325:u8)
                n118 = Build Array(u8 2, w326, w325) -> (w324:u8[])
              }
              frame "关闭" {
                n119 = Split Number(x=u16 52394) -> (hi(x)=w331:u8, lo(x)=w330:u8)
                n120 = Build Array(u8 2, w331, w330) -> (w329:u8[])
              }
            }
            n121 = Bundle By Name(cluster=T6 {"ID"=0, "TimeStamp"=0, "TimeFlag"=0, "SendType"=0, "RemoteFlag"=0, "ExternFlag"=0, "DataLen"=0, "Data"=[], "Reserved"=[]} ("Send"), "ID"=w307, "RemoteFlag"=w315, "ExternFlag"=w316, "DataLen"=u8 3, "Data"=w304) -> (w314:T6)
            n122 = Build Array(w314) -> (w313:T6[])
            n123 = Unbundle By Name(w308) -> ("DevType"=w310:T5, "DevIndex"=w311:u32, "CanIndex"=w312:T4)
            n124 = call "VCI_Transmit.vi"("Buffer"=w313, "CANIndex"=w312, "DevIndex"=w311, "DevType"=w310) -> ()  [unwired: 1 in, 7 out]
          }
          event "模式_W": Value Change {
            w340 = u8 0 items=["数据帧", "遥控帧"]
            w339 = u8 0 items=["标准帧", "扩展帧"]
            # "地址"
            n125 = event-data() -> ()  [unwired: 2 out]
            n126 = property on="电机ID" class="CmbBox"() -> ("Value"=w349:string)  [unwired: 2 in, 2 out]
            n127 = Concatenate Strings("20 ", "模式") -> (w353:string)
            n128 = Scan From String(format string="%x" ("格式字符串"), input string=w349, default 1=u8 0) -> (output 1=w352:u8)  [unwired: 2 in, 3 out]
            n129 = property on="模式_回" class="CmbBox"("Value"="模式") -> ()  [unwired: 2 in, 2 out]
            n130 = call "Demo_MakeData.vi"("DataString"=w353) -> ("Data"=w336:u8[], "DataLen"=w344:u8)  [unwired: 9 out]
            n131 = Add(x=u32 16, y=w352) -> (x+y=w335:u32)
            n132 = Bundle By Name(cluster=T6 {"ID"=0, "TimeStamp"=0, "TimeFlag"=0, "SendType"=0, "RemoteFlag"=0, "ExternFlag"=0, "DataLen"=0, "Data"=[], "Reserved"=[]} ("Send"), "ID"=w335, "RemoteFlag"=w340, "ExternFlag"=w339, "DataLen"=w344, "Data"=w336) -> (w341:T6)
            n133 = Build Array(w341) -> (w342:T6[])
            n134 = Unbundle By Name(w338) -> ("DevType"=w346:T5, "DevIndex"=w345:u32, "CanIndex"=w343:T4)
            n135 = call "VCI_Transmit.vi"("Buffer"=w342, "CANIndex"=w343, "DevIndex"=w345, "DevType"=w346) -> ()  [unwired: 1 in, 7 out]
          }
          event "模式_R": Value Change {
            w373 = u8 0 items=["数据帧", "遥控帧"]
            w374 = u8 0 items=["标准帧", "扩展帧"]
            # "地址"
            n136 = event-data() -> ()  [unwired: 2 out]
            n137 = property on="电机ID" class="CmbBox"() -> ("Value"=w364:string)  [unwired: 2 in, 2 out]
            n138 = Scan From String(format string="%x" ("格式字符串"), input string=w364, default 1=u8 0) -> (output 1=w361:u8)  [unwired: 2 in, 3 out]
            n139 = call "Demo_MakeData.vi"("DataString"="20 ") -> ("Data"=w358:u8[], "DataLen"=w369:u8)  [unwired: 9 out]
            n140 = Add(x=u32 48, y=w361) -> (x+y=w357:u32)
            n141 = Bundle By Name(cluster=T6 {"ID"=0, "TimeStamp"=0, "TimeFlag"=0, "SendType"=0, "RemoteFlag"=0, "ExternFlag"=0, "DataLen"=0, "Data"=[], "Reserved"=[]} ("Send"), "ID"=w357, "RemoteFlag"=w373, "ExternFlag"=w374, "DataLen"=w369, "Data"=w358) -> (w372:T6)
            n142 = Build Array(w372) -> (w371:T6[])
            n143 = Unbundle By Name(w360) -> ("DevType"=w367:T5, "DevIndex"=w368:u32, "CanIndex"=w370:T4)
            n144 = call "VCI_Transmit.vi"("Buffer"=w371, "CANIndex"=w370, "DevIndex"=w368, "DevType"=w367) -> ()  [unwired: 1 in, 7 out]
          }
          event "设定位置_W": Value Change {
            w390 = u8 0 items=["数据帧", "遥控帧"]
            w389 = u8 0 items=["标准帧", "扩展帧"]
            # "索引地址"
            n145 = event-data() -> ()  [unwired: 2 out]
            n146 = property on="电机ID" class="CmbBox"() -> ("Value"=w398:string)  [unwired: 2 in, 2 out]
            n147 = Multiply ("乘")(x="设定位置", y=u16 256) -> (x*y=w382:i16)
            n148 = Scan From String(format string="%x" ("格式字符串"), input string=w398, default 1=u8 0) -> (output 1=w401:u8)  [unwired: 2 in, 3 out]
            n149 = Split Number(x=w382) -> (hi(x)=w381:u8, lo(x)=w380:u8)
            n150 = Add(x=u32 16, y=w401) -> (x+y=w378:u32)
            n151 = Build Array(u8 64, w381, w380) -> (w379:u8[])
            n152 = Bundle By Name(cluster=T6 {"ID"=0, "TimeStamp"=0, "TimeFlag"=0, "SendType"=0, "RemoteFlag"=0, "ExternFlag"=0, "DataLen"=0, "Data"=[], "Reserved"=[]} ("Send"), "ID"=w378, "RemoteFlag"=w390, "ExternFlag"=w389, "DataLen"=u8 3, "Data"=w379) -> (w391:T6)
            n153 = Build Array(w391) -> (w392:T6[])
            n154 = Unbundle By Name(w388) -> ("DevType"=w395:T5, "DevIndex"=w394:u32, "CanIndex"=w393:T4)
            n155 = call "VCI_Transmit.vi"("Buffer"=w392, "CANIndex"=w393, "DevIndex"=w394, "DevType"=w395) -> ()  [unwired: 1 in, 7 out]
          }
          event "设定速度_W": Value Change {
            w423 = u8 0 items=["数据帧", "遥控帧"]
            w424 = u8 0 items=["标准帧", "扩展帧"]
            # "索引地址"
            n156 = event-data() -> ()  [unwired: 2 out]
            n157 = property on="电机ID" class="CmbBox"() -> ("Value"=w415:string)  [unwired: 2 in, 2 out]
            n158 = Multiply ("乘")(x="设定速度", y=i16 1) -> (x*y=w408:i16)
            n159 = Scan From String(format string="%x" ("格式字符串"), input string=w415, default 1=u8 0) -> (output 1=w412:u8)  [unwired: 2 in, 3 out]
            n160 = Split Number(x=w408) -> (hi(x)=w407:u8, lo(x)=w406:u8)
            n161 = Add(x=u32 16, y=w412) -> (x+y=w404:u32)
            n162 = Build Array(u8 65, w407, w406) -> (w405:u8[])
            n163 = Bundle By Name(cluster=T6 {"ID"=0, "TimeStamp"=0, "TimeFlag"=0, "SendType"=0, "RemoteFlag"=0, "ExternFlag"=0, "DataLen"=0, "Data"=[], "Reserved"=[]} ("Send"), "ID"=w404, "RemoteFlag"=w423, "ExternFlag"=w424, "DataLen"=u8 3, "Data"=w405) -> (w422:T6)
            n164 = Build Array(w422) -> (w421:T6[])
            n165 = Unbundle By Name(w411) -> ("DevType"=w418:T5, "DevIndex"=w419:u32, "CanIndex"=w420:T4)
            n166 = call "VCI_Transmit.vi"("Buffer"=w421, "CANIndex"=w420, "DevIndex"=w419, "DevType"=w418) -> ()  [unwired: 1 in, 7 out]
          }
          event "设定电流_W": Value Change {
            w442 = u8 0 items=["数据帧", "遥控帧"]
            w441 = u8 0 items=["标准帧", "扩展帧"]
            # "索引地址"
            n167 = event-data() -> ()  [unwired: 2 out]
            n168 = property on="电机ID" class="CmbBox"() -> ("Value"=w450:string)  [unwired: 2 in, 2 out]
            n169 = Multiply ("乘")(x="设定电流", y=i16 256) -> (x*y=w434:i16)
            n170 = Scan From String(format string="%x" ("格式字符串"), input string=w450, default 1=u8 0) -> (output 1=w453:u8)  [unwired: 2 in, 3 out]
            n171 = Split Number(x=w434) -> (hi(x)=w433:u8, lo(x)=w432:u8)
            n172 = Add(x=u32 16, y=w453) -> (x+y=w430:u32)
            n173 = Build Array(u8 66, w433, w432) -> (w431:u8[])
            n174 = Bundle By Name(cluster=T6 {"ID"=0, "TimeStamp"=0, "TimeFlag"=0, "SendType"=0, "RemoteFlag"=0, "ExternFlag"=0, "DataLen"=0, "Data"=[], "Reserved"=[]} ("Send"), "ID"=w430, "RemoteFlag"=w442, "ExternFlag"=w441, "DataLen"=u8 3, "Data"=w431) -> (w443:T6)
            n175 = Build Array(w443) -> (w444:T6[])
            n176 = Unbundle By Name(w437) -> ("DevType"=w447:T5, "DevIndex"=w446:u32, "CanIndex"=w445:T4)
            n177 = call "VCI_Transmit.vi"("Buffer"=w444, "CANIndex"=w445, "DevIndex"=w446, "DevType"=w447) -> ()  [unwired: 1 in, 7 out]
          }
          event "电流环KP_W": Value Change {
            w472 = u8 0 items=["数据帧", "遥控帧"]
            w473 = u8 0 items=["标准帧", "扩展帧"]
            # "索引地址"
            n178 = event-data() -> ()  [unwired: 2 out]
            n179 = property on="电机ID" class="CmbBox"() -> ("Value"=w464:string)  [unwired: 2 in, 2 out]
            n180 = Multiply ("乘")(x="电流环KP", y=u16 256) -> (x*y=w477:u16)
            n181 = Scan From String(format string="%x" ("格式字符串"), input string=w464, default 1=u8 0) -> (output 1=w461:u8)  [unwired: 2 in, 3 out]
            n182 = Split Number(x=w477) -> (hi(x)=w478:u8, lo(x)=w479:u8)
            n183 = Add(x=u32 16, y=w461) -> (x+y=w456:u32)
            n184 = Build Array(u8 81, w478, w479) -> (w457:u8[])
            n185 = Bundle By Name(cluster=T6 {"ID"=0, "TimeStamp"=0, "TimeFlag"=0, "SendType"=0, "RemoteFlag"=0, "ExternFlag"=0, "DataLen"=0, "Data"=[], "Reserved"=[]} ("Send"), "ID"=w456, "RemoteFlag"=w472, "ExternFlag"=w473, "DataLen"=u8 3, "Data"=w457) -> (w471:T6)
            n186 = Build Array(w471) -> (w470:T6[])
            n187 = Unbundle By Name(w460) -> ("DevType"=w467:T5, "DevIndex"=w468:u32, "CanIndex"=w469:T4)
            n188 = call "VCI_Transmit.vi"("Buffer"=w470, "CANIndex"=w469, "DevIndex"=w468, "DevType"=w467) -> ()  [unwired: 1 in, 7 out]
          }
          event "电流环KI_W": Value Change {
            w494 = u8 0 items=["数据帧", "遥控帧"]
            w493 = u8 0 items=["标准帧", "扩展帧"]
            # "索引地址"
            n189 = event-data() -> ()  [unwired: 2 out]
            n190 = property on="电机ID" class="CmbBox"() -> ("Value"=w502:string)  [unwired: 2 in, 2 out]
            n191 = Multiply ("乘")(x="电流环KI", y=u16 256) -> (x*y=w489:u16)
            n192 = Scan From String(format string="%x" ("格式字符串"), input string=w502, default 1=u8 0) -> (output 1=w505:u8)  [unwired: 2 in, 3 out]
            n193 = Split Number(x=w489) -> (hi(x)=w488:u8, lo(x)=w487:u8)
            n194 = Add(x=u32 16, y=w505) -> (x+y=w482:u32)
            n195 = Build Array(u8 82, w488, w487) -> (w483:u8[])
            n196 = Bundle By Name(cluster=T6 {"ID"=0, "TimeStamp"=0, "TimeFlag"=0, "SendType"=0, "RemoteFlag"=0, "ExternFlag"=0, "DataLen"=0, "Data"=[], "Reserved"=[]} ("Send"), "ID"=w482, "RemoteFlag"=w494, "ExternFlag"=w493, "DataLen"=u8 3, "Data"=w483) -> (w495:T6)
            n197 = Build Array(w495) -> (w496:T6[])
            n198 = Unbundle By Name(w486) -> ("DevType"=w499:T5, "DevIndex"=w498:u32, "CanIndex"=w497:T4)
            n199 = call "VCI_Transmit.vi"("Buffer"=w496, "CANIndex"=w497, "DevIndex"=w498, "DevType"=w499) -> ()  [unwired: 1 in, 7 out]
          }
          event "速度环KP_W": Value Change {
            w520 = u8 0 items=["数据帧", "遥控帧"]
            w519 = u8 0 items=["标准帧", "扩展帧"]
            # "索引地址"
            n200 = event-data() -> ()  [unwired: 2 out]
            n201 = property on="电机ID" class="CmbBox"() -> ("Value"=w528:string)  [unwired: 2 in, 2 out]
            n202 = Multiply ("乘")(x="速度环KP", y=u16 256) -> (x*y=w515:u16)
            n203 = Scan From String(format string="%x" ("格式字符串"), input string=w528, default 1=u8 0) -> (output 1=w531:u8)  [unwired: 2 in, 3 out]
            n204 = Split Number(x=w515) -> (hi(x)=w514:u8, lo(x)=w513:u8)
            n205 = Add(x=u32 16, y=w531) -> (x+y=w508:u32)
            n206 = Build Array(u8 83, w514, w513) -> (w509:u8[])
            n207 = Bundle By Name(cluster=T6 {"ID"=0, "TimeStamp"=0, "TimeFlag"=0, "SendType"=0, "RemoteFlag"=0, "ExternFlag"=0, "DataLen"=0, "Data"=[], "Reserved"=[]} ("Send"), "ID"=w508, "RemoteFlag"=w520, "ExternFlag"=w519, "DataLen"=u8 3, "Data"=w509) -> (w521:T6)
            n208 = Build Array(w521) -> (w522:T6[])
            n209 = Unbundle By Name(w512) -> ("DevType"=w525:T5, "DevIndex"=w524:u32, "CanIndex"=w523:T4)
            n210 = call "VCI_Transmit.vi"("Buffer"=w522, "CANIndex"=w523, "DevIndex"=w524, "DevType"=w525) -> ()  [unwired: 1 in, 7 out]
          }
          event "速度环KI_W": Value Change {
            w550 = u8 0 items=["数据帧", "遥控帧"]
            w551 = u8 0 items=["标准帧", "扩展帧"]
            # "索引地址"
            n211 = event-data() -> ()  [unwired: 2 out]
            n212 = property on="电机ID" class="CmbBox"() -> ("Value"=w542:string)  [unwired: 2 in, 2 out]
            n213 = Multiply ("乘")(x="速度环KI", y=u16 256) -> (x*y=w555:u16)
            n214 = Scan From String(format string="%x" ("格式字符串"), input string=w542, default 1=u8 0) -> (output 1=w539:u8)  [unwired: 2 in, 3 out]
            n215 = Split Number(x=w555) -> (hi(x)=w556:u8, lo(x)=w557:u8)
            n216 = Add(x=u32 16, y=w539) -> (x+y=w534:u32)
            n217 = Build Array(u8 84, w556, w557) -> (w535:u8[])
            n218 = Bundle By Name(cluster=T6 {"ID"=0, "TimeStamp"=0, "TimeFlag"=0, "SendType"=0, "RemoteFlag"=0, "ExternFlag"=0, "DataLen"=0, "Data"=[], "Reserved"=[]} ("Send"), "ID"=w534, "RemoteFlag"=w550, "ExternFlag"=w551, "DataLen"=u8 3, "Data"=w535) -> (w549:T6)
            n219 = Build Array(w549) -> (w548:T6[])
            n220 = Unbundle By Name(w538) -> ("DevType"=w545:T5, "DevIndex"=w546:u32, "CanIndex"=w547:T4)
            n221 = call "VCI_Transmit.vi"("Buffer"=w548, "CANIndex"=w547, "DevIndex"=w546, "DevType"=w545) -> ()  [unwired: 1 in, 7 out]
          }
          event "加速度_W": Value Change {
            w572 = u8 0 items=["数据帧", "遥控帧"]
            w571 = u8 0 items=["标准帧", "扩展帧"]
            # "索引地址"
            n222 = event-data() -> ()  [unwired: 2 out]
            n223 = property on="电机ID" class="CmbBox"() -> ("Value"=w580:string)  [unwired: 2 in, 2 out]
            n224 = Multiply ("乘")(x="加速度", y=u16 8) -> (x*y=w567:u16)
            n225 = Scan From String(format string="%x" ("格式字符串"), input string=w580, default 1=u8 0) -> (output 1=w583:u8)  [unwired: 2 in, 3 out]
            n226 = Split Number(x=w567) -> (hi(x)=w566:u8, lo(x)=w565:u8)
            n227 = Add(x=u32 16, y=w583) -> (x+y=w560:u32)
            n228 = Build Array(u8 85, w566, w565) -> (w561:u8[])
            n229 = Bundle By Name(cluster=T6 {"ID"=0, "TimeStamp"=0, "TimeFlag"=0, "SendType"=0, "RemoteFlag"=0, "ExternFlag"=0, "DataLen"=0, "Data"=[], "Reserved"=[]} ("Send"), "ID"=w560, "RemoteFlag"=w572, "ExternFlag"=w571, "DataLen"=u8 3, "Data"=w561) -> (w573:T6)
            n230 = Build Array(w573) -> (w574:T6[])
            n231 = Unbundle By Name(w564) -> ("DevType"=w577:T5, "DevIndex"=w576:u32, "CanIndex"=w575:T4)
            n232 = call "VCI_Transmit.vi"("Buffer"=w574, "CANIndex"=w575, "DevIndex"=w576, "DevType"=w577) -> ()  [unwired: 1 in, 7 out]
          }
          event "AI_K0_W": Value Change {
            w596 = u8 0 items=["数据帧", "遥控帧"]
            w595 = u8 0 items=["标准帧", "扩展帧"]
            # "索引地址"
            n233 = event-data() -> ()  [unwired: 2 out]
            n234 = property on="电机ID" class="CmbBox"() -> ("Value"=w604:string)  [unwired: 2 in, 2 out]
            n235 = Scan From String(format string="%x" ("格式字符串"), input string=w604, default 1=u8 0) -> (output 1=w607:u8)  [unwired: 2 in, 3 out]
            n236 = Split Number(x="A电流零偏") -> (hi(x)=w592:u8, lo(x)=w591:u8)
            n237 = Add(x=u32 16, y=w607) -> (x+y=w586:u32)
            n238 = Build Array(u8 90, w592, w591) -> (w587:u8[])
            n239 = Bundle By Name(cluster=T6 {"ID"=0, "TimeStamp"=0, "TimeFlag"=0, "SendType"=0, "RemoteFlag"=0, "ExternFlag"=0, "DataLen"=0, "Data"=[], "Reserved"=[]} ("Send"), "ID"=w586, "RemoteFlag"=w596, "ExternFlag"=w595, "DataLen"=u8 3, "Data"=w587) -> (w597:T6)
            n240 = Build Array(w597) -> (w598:T6[])
            n241 = Unbundle By Name(w590) -> ("DevType"=w601:T5, "DevIndex"=w600:u32, "CanIndex"=w599:T4)
            n242 = call "VCI_Transmit.vi"("Buffer"=w598, "CANIndex"=w599, "DevIndex"=w600, "DevType"=w601) -> ()  [unwired: 1 in, 7 out]
          }
          event "BI_K0_W": Value Change {
            w620 = u8 0 items=["数据帧", "遥控帧"]
            w619 = u8 0 items=["标准帧", "扩展帧"]
            # "索引地址"
            n243 = event-data() -> ()  [unwired: 2 out]
            n244 = property on="电机ID" class="CmbBox"() -> ("Value"=w628:string)  [unwired: 2 in, 2 out]
            n245 = Scan From String(format string="%x" ("格式字符串"), input string=w628, default 1=u8 0) -> (output 1=w631:u8)  [unwired: 2 in, 3 out]
            n246 = Split Number(x="B电流零偏") -> (hi(x)=w616:u8, lo(x)=w615:u8)
            n247 = Add(x=u32 16, y=w631) -> (x+y=w610:u32)
            n248 = Build Array(u8 91, w616, w615) -> (w611:u8[])
            n249 = Bundle By Name(cluster=T6 {"ID"=0, "TimeStamp"=0, "TimeFlag"=0, "SendType"=0, "RemoteFlag"=0, "ExternFlag"=0, "DataLen"=0, "Data"=[], "Reserved"=[]} ("Send"), "ID"=w610, "RemoteFlag"=w620, "ExternFlag"=w619, "DataLen"=u8 3, "Data"=w611) -> (w621:T6)
            n250 = Build Array(w621) -> (w622:T6[])
            n251 = Unbundle By Name(w614) -> ("DevType"=w625:T5, "DevIndex"=w624:u32, "CanIndex"=w623:T4)
            n252 = call "VCI_Transmit.vi"("Buffer"=w622, "CANIndex"=w623, "DevIndex"=w624, "DevType"=w625) -> ()  [unwired: 1 in, 7 out]
          }
          event "CI_K0_W": Value Change {
            w644 = u8 0 items=["数据帧", "遥控帧"]
            w643 = u8 0 items=["标准帧", "扩展帧"]
            # "索引地址"
            n253 = event-data() -> ()  [unwired: 2 out]
            n254 = property on="电机ID" class="CmbBox"() -> ("Value"=w652:string)  [unwired: 2 in, 2 out]
            n255 = Scan From String(format string="%x" ("格式字符串"), input string=w652, default 1=u8 0) -> (output 1=w655:u8)  [unwired: 2 in, 3 out]
            n256 = Split Number(x="C电流零偏") -> (hi(x)=w640:u8, lo(x)=w639:u8)
            n257 = Add(x=u32 16, y=w655) -> (x+y=w634:u32)
            n258 = Build Array(u8 92, w640, w639) -> (w635:u8[])
            n259 = Bundle By Name(cluster=T6 {"ID"=0, "TimeStamp"=0, "TimeFlag"=0, "SendType"=0, "RemoteFlag"=0, "ExternFlag"=0, "DataLen"=0, "Data"=[], "Reserved"=[]} ("Send"), "ID"=w634, "RemoteFlag"=w644, "ExternFlag"=w643, "DataLen"=u8 3, "Data"=w635) -> (w645:T6)
            n260 = Build Array(w645) -> (w646:T6[])
            n261 = Unbundle By Name(w638) -> ("DevType"=w649:T5, "DevIndex"=w648:u32, "CanIndex"=w647:T4)
            n262 = call "VCI_Transmit.vi"("Buffer"=w646, "CANIndex"=w647, "DevIndex"=w648, "DevType"=w649) -> ()  [unwired: 1 in, 7 out]
          }
          event "DATA_SAVE_W": Value Change {
            w674 = u8 0 items=["数据帧", "遥控帧"]
            w675 = u8 0 items=["标准帧", "扩展帧"]
            # "地址"
            n263 = event-data() -> ()  [unwired: 2 out]
            n264 = property on="电机ID" class="CmbBox"() -> ("Value"=w665:string)  [unwired: 2 in, 2 out]
            n265 = Scan From String(format string="%x" ("格式字符串"), input string=w665, default 1=u8 0) -> (output 1=w662:u8)  [unwired: 2 in, 3 out]
            n266 = call "Demo_MakeData.vi"("DataString"="50") -> ("Data"=w659:u8[], "DataLen"=w670:u8)  [unwired: 9 out]
            n267 = Add(x=u32 16, y=w662) -> (x+y=w658:u32)
            n268 = Bundle By Name(cluster=T6 {"ID"=0, "TimeStamp"=0, "TimeFlag"=0, "SendType"=0, "RemoteFlag"=0, "ExternFlag"=0, "DataLen"=0, "Data"=[], "Reserved"=[]} ("Send"), "ID"=w658, "RemoteFlag"=w674, "ExternFlag"=w675, "DataLen"=w670, "Data"=w659) -> (w673:T6)
            n269 = Build Array(w673) -> (w672:T6[])
            n270 = Unbundle By Name(w661) -> ("DevType"=w668:T5, "DevIndex"=w669:u32, "CanIndex"=w671:T4)
            n271 = call "VCI_Transmit.vi"("Buffer"=w672, "CANIndex"=w671, "DevIndex"=w669, "DevType"=w668) -> ()  [unwired: 1 in, 7 out]
          }
          event "设定位置_R": Value Change {
            w685 = u8 0 items=["数据帧", "遥控帧"]
            w684 = u8 0 items=["标准帧", "扩展帧"]
            # "地址"
            n272 = event-data() -> ()  [unwired: 2 out]
            n273 = property on="电机ID" class="CmbBox"() -> ("Value"=w694:string)  [unwired: 2 in, 2 out]
            n274 = Scan From String(format string="%x" ("格式字符串"), input string=w694, default 1=u8 0) -> (output 1=w697:u8)  [unwired: 2 in, 3 out]
            n275 = call "Demo_MakeData.vi"("DataString"="40 ") -> ("Data"=w680:u8[], "DataLen"=w689:u8)  [unwired: 9 out]
            n276 = Add(x=u32 48, y=w697) -> (x+y=w679:u32)
            n277 = Bundle By Name(cluster=T6 {"ID"=0, "TimeStamp"=0, "TimeFlag"=0, "SendType"=0, "RemoteFlag"=0, "ExternFlag"=0, "DataLen"=0, "Data"=[], "Reserved"=[]} ("Send"), "ID"=w679, "RemoteFlag"=w685, "ExternFlag"=w684, "DataLen"=w689, "Data"=w680) -> (w686:T6)
            n278 = Build Array(w686) -> (w687:T6[])
            n279 = Unbundle By Name(w682) -> ("DevType"=w691:T5, "DevIndex"=w690:u32, "CanIndex"=w688:T4)
            n280 = call "VCI_Transmit.vi"("Buffer"=w687, "CANIndex"=w688, "DevIndex"=w690, "DevType"=w691) -> ()  [unwired: 1 in, 7 out]
          }
          event "设定速度_R": Value Change {
            w716 = u8 0 items=["数据帧", "遥控帧"]
            w717 = u8 0 items=["标准帧", "扩展帧"]
            # "地址"
            n281 = event-data() -> ()  [unwired: 2 out]
            n282 = property on="电机ID" class="CmbBox"() -> ("Value"=w707:string)  [unwired: 2 in, 2 out]
            n283 = Scan From String(format string="%x" ("格式字符串"), input string=w707, default 1=u8 0) -> (output 1=w704:u8)  [unwired: 2 in, 3 out]
            n284 = call "Demo_MakeData.vi"("DataString"="41 ") -> ("Data"=w701:u8[], "DataLen"=w712:u8)  [unwired: 9 out]
            n285 = Add(x=u32 48, y=w704) -> (x+y=w700:u32)
            n286 = Bundle By Name(cluster=T6 {"ID"=0, "TimeStamp"=0, "TimeFlag"=0, "SendType"=0, "RemoteFlag"=0, "ExternFlag"=0, "DataLen"=0, "Data"=[], "Reserved"=[]} ("Send"), "ID"=w700, "RemoteFlag"=w716, "ExternFlag"=w717, "DataLen"=w712, "Data"=w701) -> (w715:T6)
            n287 = Build Array(w715) -> (w714:T6[])
            n288 = Unbundle By Name(w703) -> ("DevType"=w710:T5, "DevIndex"=w711:u32, "CanIndex"=w713:T4)
            n289 = call "VCI_Transmit.vi"("Buffer"=w714, "CANIndex"=w713, "DevIndex"=w711, "DevType"=w710) -> ()  [unwired: 1 in, 7 out]
          }
          event "设定电流_R": Value Change {
            w737 = u8 0 items=["数据帧", "遥控帧"]
            w738 = u8 0 items=["标准帧", "扩展帧"]
            # "地址"
            n290 = event-data() -> ()  [unwired: 2 out]
            n291 = property on="电机ID" class="CmbBox"() -> ("Value"=w728:string)  [unwired: 2 in, 2 out]
            n292 = Scan From String(format string="%x" ("格式字符串"), input string=w728, default 1=u8 0) -> (output 1=w725:u8)  [unwired: 2 in, 3 out]
            n293 = call "Demo_MakeData.vi"("DataString"="42 ") -> ("Data"=w722:u8[], "DataLen"=w733:u8)  [unwired: 9 out]
            n294 = Add(x=u32 48, y=w725) -> (x+y=w721:u32)
            n295 = Bundle By Name(cluster=T6 {"ID"=0, "TimeStamp"=0, "TimeFlag"=0, "SendType"=0, "RemoteFlag"=0, "ExternFlag"=0, "DataLen"=0, "Data"=[], "Reserved"=[]} ("Send"), "ID"=w721, "RemoteFlag"=w737, "ExternFlag"=w738, "DataLen"=w733, "Data"=w722) -> (w736:T6)
            n296 = Build Array(w736) -> (w735:T6[])
            n297 = Unbundle By Name(w724) -> ("DevType"=w731:T5, "DevIndex"=w732:u32, "CanIndex"=w734:T4)
            n298 = call "VCI_Transmit.vi"("Buffer"=w735, "CANIndex"=w734, "DevIndex"=w732, "DevType"=w731) -> ()  [unwired: 1 in, 7 out]
          }
          event "电流环KP_R": Value Change {
            w758 = u8 0 items=["数据帧", "遥控帧"]
            w759 = u8 0 items=["标准帧", "扩展帧"]
            # "地址"
            n299 = event-data() -> ()  [unwired: 2 out]
            n300 = property on="电机ID" class="CmbBox"() -> ("Value"=w749:string)  [unwired: 2 in, 2 out]
            n301 = Scan From String(format string="%x" ("格式字符串"), input string=w749, default 1=u8 0) -> (output 1=w746:u8)  [unwired: 2 in, 3 out]
            n302 = call "Demo_MakeData.vi"("DataString"="51 ") -> ("Data"=w743:u8[], "DataLen"=w754:u8)  [unwired: 9 out]
            n303 = Add(x=u32 48, y=w746) -> (x+y=w742:u32)
            n304 = Bundle By Name(cluster=T6 {"ID"=0, "TimeStamp"=0, "TimeFlag"=0, "SendType"=0, "RemoteFlag"=0, "ExternFlag"=0, "DataLen"=0, "Data"=[], "Reserved"=[]} ("Send"), "ID"=w742, "RemoteFlag"=w758, "ExternFlag"=w759, "DataLen"=w754, "Data"=w743) -> (w757:T6)
            n305 = Build Array(w757) -> (w756:T6[])
            n306 = Unbundle By Name(w745) -> ("DevType"=w752:T5, "DevIndex"=w753:u32, "CanIndex"=w755:T4)
            n307 = call "VCI_Transmit.vi"("Buffer"=w756, "CANIndex"=w755, "DevIndex"=w753, "DevType"=w752) -> ()  [unwired: 1 in, 7 out]
          }
          event "电流环KI_R": Value Change {
            w779 = u8 0 items=["数据帧", "遥控帧"]
            w780 = u8 0 items=["标准帧", "扩展帧"]
            # "地址"
            n308 = event-data() -> ()  [unwired: 2 out]
            n309 = property on="电机ID" class="CmbBox"() -> ("Value"=w770:string)  [unwired: 2 in, 2 out]
            n310 = Scan From String(format string="%x" ("格式字符串"), input string=w770, default 1=u8 0) -> (output 1=w767:u8)  [unwired: 2 in, 3 out]
            n311 = call "Demo_MakeData.vi"("DataString"="52 ") -> ("Data"=w764:u8[], "DataLen"=w775:u8)  [unwired: 9 out]
            n312 = Add(x=u32 48, y=w767) -> (x+y=w763:u32)
            n313 = Bundle By Name(cluster=T6 {"ID"=0, "TimeStamp"=0, "TimeFlag"=0, "SendType"=0, "RemoteFlag"=0, "ExternFlag"=0, "DataLen"=0, "Data"=[], "Reserved"=[]} ("Send"), "ID"=w763, "RemoteFlag"=w779, "ExternFlag"=w780, "DataLen"=w775, "Data"=w764) -> (w778:T6)
            n314 = Build Array(w778) -> (w777:T6[])
            n315 = Unbundle By Name(w766) -> ("DevType"=w773:T5, "DevIndex"=w774:u32, "CanIndex"=w776:T4)
            n316 = call "VCI_Transmit.vi"("Buffer"=w777, "CANIndex"=w776, "DevIndex"=w774, "DevType"=w773) -> ()  [unwired: 1 in, 7 out]
          }
          event "速度环KP_R": Value Change {
            w790 = u8 0 items=["数据帧", "遥控帧"]
            w789 = u8 0 items=["标准帧", "扩展帧"]
            # "地址"
            n317 = event-data() -> ()  [unwired: 2 out]
            n318 = property on="电机ID" class="CmbBox"() -> ("Value"=w799:string)  [unwired: 2 in, 2 out]
            n319 = Scan From String(format string="%x" ("格式字符串"), input string=w799, default 1=u8 0) -> (output 1=w802:u8)  [unwired: 2 in, 3 out]
            n320 = call "Demo_MakeData.vi"("DataString"="53 ") -> ("Data"=w785:u8[], "DataLen"=w794:u8)  [unwired: 9 out]
            n321 = Add(x=u32 48, y=w802) -> (x+y=w784:u32)
            n322 = Bundle By Name(cluster=T6 {"ID"=0, "TimeStamp"=0, "TimeFlag"=0, "SendType"=0, "RemoteFlag"=0, "ExternFlag"=0, "DataLen"=0, "Data"=[], "Reserved"=[]} ("Send"), "ID"=w784, "RemoteFlag"=w790, "ExternFlag"=w789, "DataLen"=w794, "Data"=w785) -> (w791:T6)
            n323 = Build Array(w791) -> (w792:T6[])
            n324 = Unbundle By Name(w787) -> ("DevType"=w796:T5, "DevIndex"=w795:u32, "CanIndex"=w793:T4)
            n325 = call "VCI_Transmit.vi"("Buffer"=w792, "CANIndex"=w793, "DevIndex"=w795, "DevType"=w796) -> ()  [unwired: 1 in, 7 out]
          }
          event "速度环KI_R": Value Change {
            w811 = u8 0 items=["数据帧", "遥控帧"]
            w810 = u8 0 items=["标准帧", "扩展帧"]
            # "地址"
            n326 = event-data() -> ()  [unwired: 2 out]
            n327 = property on="电机ID" class="CmbBox"() -> ("Value"=w820:string)  [unwired: 2 in, 2 out]
            n328 = Scan From String(format string="%x" ("格式字符串"), input string=w820, default 1=u8 0) -> (output 1=w823:u8)  [unwired: 2 in, 3 out]
            n329 = call "Demo_MakeData.vi"("DataString"="54 ") -> ("Data"=w806:u8[], "DataLen"=w815:u8)  [unwired: 9 out]
            n330 = Add(x=u32 48, y=w823) -> (x+y=w805:u32)
            n331 = Bundle By Name(cluster=T6 {"ID"=0, "TimeStamp"=0, "TimeFlag"=0, "SendType"=0, "RemoteFlag"=0, "ExternFlag"=0, "DataLen"=0, "Data"=[], "Reserved"=[]} ("Send"), "ID"=w805, "RemoteFlag"=w811, "ExternFlag"=w810, "DataLen"=w815, "Data"=w806) -> (w812:T6)
            n332 = Build Array(w812) -> (w813:T6[])
            n333 = Unbundle By Name(w808) -> ("DevType"=w817:T5, "DevIndex"=w816:u32, "CanIndex"=w814:T4)
            n334 = call "VCI_Transmit.vi"("Buffer"=w813, "CANIndex"=w814, "DevIndex"=w816, "DevType"=w817) -> ()  [unwired: 1 in, 7 out]
          }
          event "加速度_R": Value Change {
            w842 = u8 0 items=["数据帧", "遥控帧"]
            w843 = u8 0 items=["标准帧", "扩展帧"]
            # "地址"
            n335 = event-data() -> ()  [unwired: 2 out]
            n336 = property on="电机ID" class="CmbBox"() -> ("Value"=w833:string)  [unwired: 2 in, 2 out]
            n337 = Scan From String(format string="%x" ("格式字符串"), input string=w833, default 1=u8 0) -> (output 1=w830:u8)  [unwired: 2 in, 3 out]
            n338 = call "Demo_MakeData.vi"("DataString"="55") -> ("Data"=w827:u8[], "DataLen"=w838:u8)  [unwired: 9 out]
            n339 = Add(x=u32 48, y=w830) -> (x+y=w826:u32)
            n340 = Bundle By Name(cluster=T6 {"ID"=0, "TimeStamp"=0, "TimeFlag"=0, "SendType"=0, "RemoteFlag"=0, "ExternFlag"=0, "DataLen"=0, "Data"=[], "Reserved"=[]} ("Send"), "ID"=w826, "RemoteFlag"=w842, "ExternFlag"=w843, "DataLen"=w838, "Data"=w827) -> (w841:T6)
            n341 = Build Array(w841) -> (w840:T6[])
            n342 = Unbundle By Name(w829) -> ("DevType"=w836:T5, "DevIndex"=w837:u32, "CanIndex"=w839:T4)
            n343 = call "VCI_Transmit.vi"("Buffer"=w840, "CANIndex"=w839, "DevIndex"=w837, "DevType"=w836) -> ()  [unwired: 1 in, 7 out]
          }
          event "AI_K0_R": Value Change {
            w853 = u8 0 items=["数据帧", "遥控帧"]
            w852 = u8 0 items=["标准帧", "扩展帧"]
            # "地址"
            n344 = event-data() -> ()  [unwired: 2 out]
            n345 = property on="电机ID" class="CmbBox"() -> ("Value"=w862:string)  [unwired: 2 in, 2 out]
            n346 = Scan From String(format string="%x" ("格式字符串"), input string=w862, default 1=u8 0) -> (output 1=w865:u8)  [unwired: 2 in, 3 out]
            n347 = call "Demo_MakeData.vi"("DataString"="5A") -> ("Data"=w848:u8[], "DataLen"=w857:u8)  [unwired: 9 out]
            n348 = Add(x=u32 48, y=w865) -> (x+y=w847:u32)
            n349 = Bundle By Name(cluster=T6 {"ID"=0, "TimeStamp"=0, "TimeFlag"=0, "SendType"=0, "RemoteFlag"=0, "ExternFlag"=0, "DataLen"=0, "Data"=[], "Reserved"=[]} ("Send"), "ID"=w847, "RemoteFlag"=w853, "ExternFlag"=w852, "DataLen"=w857, "Data"=w848) -> (w854:T6)
            n350 = Build Array(w854) -> (w855:T6[])
            n351 = Unbundle By Name(w850) -> ("DevType"=w859:T5, "DevIndex"=w858:u32, "CanIndex"=w856:T4)
            n352 = call "VCI_Transmit.vi"("Buffer"=w855, "CANIndex"=w856, "DevIndex"=w858, "DevType"=w859) -> ()  [unwired: 1 in, 7 out]
          }
          event "BI_K0_R": Value Change {
            w874 = u8 0 items=["数据帧", "遥控帧"]
            w873 = u8 0 items=["标准帧", "扩展帧"]
            # "地址"
            n353 = event-data() -> ()  [unwired: 2 out]
            n354 = property on="电机ID" class="CmbBox"() -> ("Value"=w883:string)  [unwired: 2 in, 2 out]
            n355 = Scan From String(format string="%x" ("格式字符串"), input string=w883, default 1=u8 0) -> (output 1=w886:u8)  [unwired: 2 in, 3 out]
            n356 = call "Demo_MakeData.vi"("DataString"="5B") -> ("Data"=w869:u8[], "DataLen"=w878:u8)  [unwired: 9 out]
            n357 = Add(x=u32 48, y=w886) -> (x+y=w868:u32)
            n358 = Bundle By Name(cluster=T6 {"ID"=0, "TimeStamp"=0, "TimeFlag"=0, "SendType"=0, "RemoteFlag"=0, "ExternFlag"=0, "DataLen"=0, "Data"=[], "Reserved"=[]} ("Send"), "ID"=w868, "RemoteFlag"=w874, "ExternFlag"=w873, "DataLen"=w878, "Data"=w869) -> (w875:T6)
            n359 = Build Array(w875) -> (w876:T6[])
            n360 = Unbundle By Name(w871) -> ("DevType"=w880:T5, "DevIndex"=w879:u32, "CanIndex"=w877:T4)
            n361 = call "VCI_Transmit.vi"("Buffer"=w876, "CANIndex"=w877, "DevIndex"=w879, "DevType"=w880) -> ()  [unwired: 1 in, 7 out]
          }
          event "CI_K0_R": Value Change {
            w895 = u8 0 items=["数据帧", "遥控帧"]
            w894 = u8 0 items=["标准帧", "扩展帧"]
            # "地址"
            n362 = event-data() -> ()  [unwired: 2 out]
            n363 = property on="电机ID" class="CmbBox"() -> ("Value"=w904:string)  [unwired: 2 in, 2 out]
            n364 = Scan From String(format string="%x" ("格式字符串"), input string=w904, default 1=u8 0) -> (output 1=w907:u8)  [unwired: 2 in, 3 out]
            n365 = call "Demo_MakeData.vi"("DataString"="5C") -> ("Data"=w890:u8[], "DataLen"=w899:u8)  [unwired: 9 out]
            n366 = Add(x=u32 48, y=w907) -> (x+y=w889:u32)
            n367 = Bundle By Name(cluster=T6 {"ID"=0, "TimeStamp"=0, "TimeFlag"=0, "SendType"=0, "RemoteFlag"=0, "ExternFlag"=0, "DataLen"=0, "Data"=[], "Reserved"=[]} ("Send"), "ID"=w889, "RemoteFlag"=w895, "ExternFlag"=w894, "DataLen"=w899, "Data"=w890) -> (w896:T6)
            n368 = Build Array(w896) -> (w897:T6[])
            n369 = Unbundle By Name(w892) -> ("DevType"=w901:T5, "DevIndex"=w900:u32, "CanIndex"=w898:T4)
            n370 = call "VCI_Transmit.vi"("Buffer"=w897, "CANIndex"=w898, "DevIndex"=w900, "DevType"=w901) -> ()  [unwired: 1 in, 7 out]
          }
          event "保存": Value Change {
            w933 = "-"
            n371 = event-data() -> ()  [unwired: 2 out]
            n372 = Get Date/Time String(want seconds? (F)=TRUE) -> (date string=w913:string, time string=w934:string)  [unwired: 2 in]
            n373 = Search and Replace String(input string=w913, search string="/", replace string="-") -> (result string=w919:string)  [unwired: 5 in, 3 out]
            n374 = Search and Replace String(input string=w934, search string=":", replace string="-") -> (result string=w931:string)  [unwired: 5 in, 3 out]
            n375 = property on="保存_S" class="Bool (严格)"() -> ("Value"=w925:bool)  [unwired: 2 in, 2 out]
            n376 = Search and Replace String(input string=w919, search string="/", replace string="-") -> (result string=w914:string)  [unwired: 5 in, 3 out]
            n377 = Search and Replace String(input string=w931, search string=":", replace string="-") -> (result string=w932:string)  [unwired: 5 in, 3 out]
            n378 = Not(x=w925) -> (.not. x?=w921:bool)
            n379 = property on="保存_S" class="Bool (严格)"("Value"=w921) -> ()  [unwired: 2 in, 2 out]
            n380 = Concatenate Strings("D:\\PMSM\\", w914, w933, w932, w933, "电机数据存储", ".txt") -> (w911:string)
            n381 = Select(t=w911, s=w921, f="") -> (s? t:f=w926:string)
            n382 = String To Path(string=w926) -> (path=w912:path)
            n383 = local write "存储路径"(w912) -> ()
          }
          event "Close": Value Change {
            w946 = T10 1 items=["OK"=1, "ERROR1"=0, "ERROR2"=-1] ("y")
            n384 = event-data() -> ()  [unwired: 2 out]
            n385 = Unbundle By Name(w950) -> ("DevType"=w949:T5, "DevIndex"=w948:u32)
            n386 = call "VCI_CloseDevice.vi"("DevIndex"=w948, "DevType"=w949) -> ("Return Val"=w947:T10)  [unwired: 1 in, 8 out]
            n387 = Equal?(x=w947, y=w946) -> (x = y?=w944:bool)
            n388 = Not(x=w944) -> (.not. x?=w940:bool)
            n389 = Bundle By Name(cluster=cluster{"CANOpen":bool} {"CANOpen"=FALSE} ("事件数据"), "CANOpen"=w940) -> (w939:cluster{"CANOpen":bool})
            n390 = Bundle By Name(cluster=w945, "Open"=w940) -> (w943:cluster{"Open":bool, "SendCnt":u32})
            n391 = local write "Open"(w940) -> ()
            n392 = Generate User Event(user event=w942, event data cluster=w939) -> ()  [unwired: 1 in, 2 out]
          }
          event User Event {
            w961 = u8 0
            w960 = u8 2
            n393 = event-data() -> ("CANOpen"=w954:bool)  [unwired: 1 out]
            "Open" <- w954
            n394 = Not(x=w954) -> (.not. x?=w955:bool)
            n395 = Select(t=w960, s=w954, f=w961) -> (s? t:f=w953:u8)
            n396 = Select(t=w961, s=w954, f=w960) -> (s? t:f=w952:u8)
            n397 = property class="VI"("Front Panel.Closeable"=w955) -> ()  [unwired: 2 in, 2 out]
            n398 = property on="Close" class="Bool"("DisabledEnum"=w952) -> ()  [unwired: 2 in, 2 out]
            n399 = property on="ID" class="DigNum (严格)"("DisabledEnum"=w952) -> ()  [unwired: 2 in, 2 out]
            n400 = property on="Data" class="Str"("DisabledEnum"=w952) -> ()  [unwired: 2 in, 2 out]
            n401 = property on="Format" class="Ring (严格)"("DisabledEnum"=w952) -> ()  [unwired: 2 in, 2 out]
            n402 = property on="Type" class="Ring (严格)"("DisabledEnum"=w952) -> ()  [unwired: 2 in, 2 out]
            n403 = property on="Send" class="Bool"("DisabledEnum"=w952) -> ()  [unwired: 2 in, 2 out]
            n404 = Select(t=enum16{"Init", "Wait", "Run", "Exit"}."Run", s=w954, f=enum16{"Init", "Wait", "Run", "Exit"}."Wait") -> (s? t:f=w957:enum16{"Init", "Wait", "Run", "Exit"})
            n405 = property on="Fliter" class="Ring (严格)"("DisabledEnum"=w953) -> ()  [unwired: 2 in, 2 out]
            n406 = property on="DevType" class="Ring (严格)"("DisabledEnum"=w953) -> ()  [unwired: 2 in, 2 out]
            n407 = property on="Channel" class="Ring (严格)"("DisabledEnum"=w953) -> ()  [unwired: 2 in, 2 out]
            n408 = property on="AccCode" class="DigNum (严格)"("DisabledEnum"=w953) -> ()  [unwired: 2 in, 2 out]
            n409 = property on="AccMask" class="DigNum (严格)"("DisabledEnum"=w953) -> ()  [unwired: 2 in, 2 out]
            n410 = property on="InitFlag" class="Ring (严格)"("DisabledEnum"=w953) -> ()  [unwired: 2 in, 2 out]
            n411 = property on="Mode" class="Ring (严格)"("DisabledEnum"=w953) -> ()  [unwired: 2 in, 2 out]
            n412 = property on="kBaudRate" class="Ring (严格)"("DisabledEnum"=w953) -> ()  [unwired: 2 in, 2 out]
            n413 = property on="电机ID_W" class="Bool"("DisabledEnum"=w952) -> ()  [unwired: 2 in, 2 out]
            n414 = property on="监测_W" class="Bool"("DisabledEnum"=w952) -> ()  [unwired: 2 in, 2 out]
            n415 = property on="模式_W" class="Bool"("DisabledEnum"=w952) -> ()  [unwired: 2 in, 2 out]
            n416 = property on="模式_R" class="Bool"("DisabledEnum"=w952) -> ()  [unwired: 2 in, 2 out]
            n417 = property on="设定位置_W" class="Bool"("DisabledEnum"=w952) -> ()  [unwired: 2 in, 2 out]
            n418 = property on="设定位置_R" class="Bool"("DisabledEnum"=w952) -> ()  [unwired: 2 in, 2 out]
            n419 = property on="设定速度_W" class="Bool"("DisabledEnum"=w952) -> ()  [unwired: 2 in, 2 out]
            n420 = property on="设定速度_R" class="Bool"("DisabledEnum"=w952) -> ()  [unwired: 2 in, 2 out]
            n421 = property on="设定电流_W" class="Bool"("DisabledEnum"=w952) -> ()  [unwired: 2 in, 2 out]
            n422 = property on="设定电流_R" class="Bool"("DisabledEnum"=w952) -> ()  [unwired: 2 in, 2 out]
            n423 = property on="保存" class="Bool"("DisabledEnum"=w952) -> ()  [unwired: 2 in, 2 out]
            n424 = property on="电流环KP_W" class="Bool"("DisabledEnum"=w952) -> ()  [unwired: 2 in, 2 out]
            n425 = property on="电流环KI_W" class="Bool"("DisabledEnum"=w952) -> ()  [unwired: 2 in, 2 out]
            n426 = property on="速度环KP_W" class="Bool"("DisabledEnum"=w952) -> ()  [unwired: 2 in, 2 out]
            n427 = property on="速度环KI_W" class="Bool"("DisabledEnum"=w952) -> ()  [unwired: 2 in, 2 out]
            n428 = property on="加速度_W" class="Bool"("DisabledEnum"=w952) -> ()  [unwired: 2 in, 2 out]
            n429 = property on="AI_K0_W" class="Bool"("DisabledEnum"=w952) -> ()  [unwired: 2 in, 2 out]
            n430 = property on="BI_K0_W" class="Bool"("DisabledEnum"=w952) -> ()  [unwired: 2 in, 2 out]
            n431 = property on="CI_K0_W" class="Bool"("DisabledEnum"=w952) -> ()  [unwired: 2 in, 2 out]
            n432 = property on="DATA_SAVE_W" class="Bool"("DisabledEnum"=w952) -> ()  [unwired: 2 in, 2 out]
            n433 = property on="监测周期_W" class="Bool"("DisabledEnum"=w952) -> ()  [unwired: 2 in, 2 out]
            n434 = property on="看门狗_W" class="Bool"("DisabledEnum"=w952) -> ()  [unwired: 2 in, 2 out]
            n435 = property on="电流环KP_R" class="Bool"("DisabledEnum"=w952) -> ()  [unwired: 2 in, 2 out]
            n436 = property on="电流环KI_R" class="Bool"("DisabledEnum"=w952) -> ()  [unwired: 2 in, 2 out]
            n437 = property on="速度环KP_R" class="Bool"("DisabledEnum"=w952) -> ()  [unwired: 2 in, 2 out]
            n438 = property on="速度环KI_R" class="Bool"("DisabledEnum"=w952) -> ()  [unwired: 2 in, 2 out]
            n439 = property on="加速度_R" class="Bool"("DisabledEnum"=w952) -> ()  [unwired: 2 in, 2 out]
            n440 = property on="AI_K0_R" class="Bool"("DisabledEnum"=w952) -> ()  [unwired: 2 in, 2 out]
            n441 = property on="BI_K0_R" class="Bool"("DisabledEnum"=w952) -> ()  [unwired: 2 in, 2 out]
            n442 = property on="CI_K0_R" class="Bool"("DisabledEnum"=w952) -> ()  [unwired: 2 in, 2 out]
            n443 = property on="监测周期_R" class="Bool"("DisabledEnum"=w952) -> ()  [unwired: 2 in, 2 out]
            n444 = property on="看门狗周期_W" class="Bool"("DisabledEnum"=w952) -> ()  [unwired: 2 in, 2 out]
            n445 = property on="看门狗周期_R" class="Bool"("DisabledEnum"=w952) -> ()  [unwired: 2 in, 2 out]
          }
        }
        "数组" <- w150
        "CAN ID" <- w149
      }
      frame "Exit" {
        n446 = Release Queue(queue=w972) -> ()  [unwired: 1 in, 4 out]
        n447 = Unregister For Events(event registration refnum=w971) -> (error out=w970:errorcluster)  [unwired: 1 in]
        n448 = Destroy User Event(user event=w969, error in=w970) -> ()  [unwired: 1 out]
        n449 = Unbundle By Name(w968) -> ("Open"=w967:bool)
        n450 = case shown="真" w967 {
          tunnel: w966 -> [_ w976]
          frame False {
          }
          frame True {
            n451 = Unbundle By Name(w976) -> ("DevType"=w975:T5, "DevIndex"=w974:u32)
            n452 = call "VCI_CloseDevice.vi"("DevIndex"=w974, "DevType"=w975) -> ()  [unwired: 1 in, 9 out]
          }
        }
        n453 = local write "RcvEnable"(FALSE ("RcvEnable")) -> ()
      }
    }
  }
  n454 = while "数据更新线程" {
    tunnel: w9 -> [w982]
    shift-right: [w977] -> _
    shift-left: u32 0 ("RecvCnt") -> [w978]
    stop <- w981 stop-if-true
    n455 = Dequeue Element(queue=w982) -> (element=w980:T7, timed out?=w979:bool, error out=w981:errorcluster)  [unwired: 2 in, 1 out]
    n456 = case shown="假" w979 {
      tunnel: w980 -> [w992 _]
      tunnel: w978 -> [w986 w1366]
      tunnel: [w985 w1366] -> w977
      frame False {
        n457 = Array To Cluster(array=w992) -> (cluster=w994:T12)
        n458 = Unbundle By Name(w994) -> ("[0]"=w993:T13)
        n459 = Increment(x=w986) -> (x+1=w985:u32)
        "sCnt" <- w985
        n460 = Unbundle By Name(w993) -> ("VCI_CAN_OBJ"=w991:T6)  [unwired: 3 out]
        n461 = Unbundle By Name(w991) -> ("ID"=w989:u32, "Data"=w990:u8[])  [unwired: 7 out]
        "CAN STD_ID" <- w989
        n462 = And(x=w989, y=u32 15) -> (x .and. y?=→"电机ID_R":u32)
        n463 = And(x=w989, y=u32 240) -> (x .and. y?=w984:u32)
        n464 = case shown="40" w984 {
          tunnel: w990 -> [_ w1000]
          frame 0, Default {
          }
          frame 64 {
            n465 = local read "存储路径"() -> (w996:path)
            n466 = local read "保存_S"() -> (w997:bool)
            n467 = Index Array(array=w1000, index=0) -> (element=w999:u8)
            n468 = case shown="5C" w999 {
              tunnel: w1000 -> [_ w1025 w1034 w1047 w1058 w1065 w1083 w1103 w1127 w1144 w1164 w1177 w1202 w1221 w1238 w1242 w1249 w1257 w1267 w1273 w1286 w1289 w1299 w1309 w1319 w1329 w1339 w1352 w1355 w1361]
              tunnel: [_ _ _ _ _ _ w1071 w1093 w1116 w1142 w1159 w1176 w1191 w1215 _ _ _ _ _ _ _ _ _ _ _ _ _ _ _ _] -> w995
              frame 0, Default {
              }
              frame 1 {
                n469 = Array To Cluster(array=w1025) -> (cluster=w1026:T14)
                n470 = Unbundle By Name(w1026) -> ("Data[1]"=w1028:u8, "Data[2]"=w1029:u8)  [unwired: 1 out]
                n471 = Join Numbers(hi=w1028, lo=w1029) -> ((hi.lo)=w1027:u16)
                n472 = To Unsigned Word Integer(number=w1027) -> (unsigned 16bit integer=→"看门狗周期_回":u16)
              }
              frame 32 {
                n473 = Array To Cluster(array=w1034) -> (cluster=w1035:T14)
                n474 = Unbundle By Name(w1035) -> ("Data[1]"=w1033:u8)  [unwired: 1 out]
                n475 = To Unsigned Byte Integer(number=w1033) -> (unsigned 8bit integer=w1030:u8)
                n476 = Number To Hexadecimal String(1:2, 2:w1030) -> (0:w1031:string)
                n477 = property on="模式_回" class="CmbBox"("Value"=w1031) -> ()  [unwired: 2 in, 2 out]
              }
              frame 33 {
                n478 = Array To Cluster(array=w1047) -> (cluster=w1049:T14)
                n479 = Unbundle By Name(w1049) -> ("Data[1]"=w1048:u8)  [unwired: 1 out]
                n480 = To Unsigned Byte Integer(number=w1048) -> (unsigned 8bit integer=w1046:u8)
                n481 = Number To Boolean Array(number=w1046) -> (Boolean array=w1045:bool[])
                n482 = Array To Cluster(array=w1045) -> (cluster=w1044:T15)
                n483 = Unbundle(w1044) -> ("Boolean array[0]"=→"warn0":bool, "Boolean array[1]"=→"warn1":bool, "Boolean array[2]"=→"高温":bool, "Boolean array[3]"=→"warn3":bool, "Boolean array[4]"=→"warn4":bool, "Boolean array[5]"=→"warn5":bool, "Boolean array[6]"=→"warn6":bool, "Boolean array[7]"=→"warn7":bool)
              }
              frame 34 {
                n484 = Array To Cluster(array=w1058) -> (cluster=w1063:T14)
                n485 = Unbundle By Name(w1063) -> ("Data[1]"=w1062:u8)  [unwired: 1 out]
                n486 = To Unsigned Byte Integer(number=w1062) -> (unsigned 8bit integer=w1061:u8)
                n487 = Number To Boolean Array(number=w1061) -> (Boolean array=w1060:bool[])
                n488 = Array To Cluster(array=w1060) -> (cluster=w1059:T15)
                n489 = Unbundle(w1059) -> ("Boolean array[0]"=→"低压":bool, "Boolean array[1]"=→"高压":bool, "Boolean array[2]"=→"高温":bool, "Boolean array[3]"=→"ERRO3":bool, "Boolean array[4]"=→"ERRO4":bool, "Boolean array[5]"=→"ERRO5":bool, "Boolean array[6]"=→"ERRO6":bool, "Boolean array[7]"=→"ERRO7":bool)
              }
              frame 35 {
                n490 = Array To Cluster(array=w1065) -> (cluster=w1066:T14)
                n491 = Unbundle By Name(w1066) -> ("Data[1]"=w1068:u8, "Data[2]"=w1069:u8)  [unwired: 1 out]
                n492 = Join Numbers(hi=w1068, lo=w1069) -> ((hi.lo)=w1067:u16)
                n493 = To Unsigned Word Integer(number=w1067) -> (unsigned 16bit integer=→"监测周期_回":u16)
              }
              frame 49 {
                w1072 = 0.0054931640625
                w1085 = 8
                n494 = Array To Cluster(array=w1083) -> (cluster=w1089:T14)
                n495 = Unbundle By Name(w1089) -> ("Data[1]"=w1077:u8, "Data[2]"=w1078:u8, "Data[3]"=w1079:u8, "Data[4]"=w1080:u8, "Data[5]"=w1076:u8, "Data[6]"=w1075:u8)  [unwired: 1 out]
                n496 = Join Numbers(hi=w1076, lo=w1075) -> ((hi.lo)=w1074:u16)
                n497 = To Unsigned Word Integer(number=w1077) -> (unsigned 16bit integer=w1092:u16)
                n498 = To Unsigned Word Integer(number=w1079) -> (unsigned 16bit integer=w1088:u16)
                n499 = To Word Integer(number=w1074) -> (16bit integer=w1073:i16)
                n500 = Rotate(1:w1092, 2:w1085) -> (0:w1091:u16)
                n501 = Rotate(1:w1088, 2:w1085) -> (0:w1087:u16)
                n502 = Add(x=w1091, y=w1078) -> (x+y=w1090:u16)
                n503 = Add(x=w1087, y=w1080) -> (x+y=w1086:u16)
                n504 = Multiply(x=w1090, y=w1072) -> (x*y=w1082:dbl)
                "机械角度" <- w1082
                n505 = Multiply(x=w1086, y=w1072) -> (x*y=w1081:dbl)
                "电气角度" <- w1081
                n506 = Divide(x=w1073, y=1.0) -> (x/y=w1070:dbl)
                "转速" <- w1070
                "电机转速" <- w1070
                n507 = Build Array(w1082, w1081, w1070) -> (w1071:dbl[])
              }
              frame 50 {
                w1104 = i16 1024
                w1105 = 8
                n508 = Array To Cluster(array=w1103) -> (cluster=w1112:T14)
                n509 = Unbundle By Name(w1112) -> ("Data[1]"=w1102:u8, "Data[2]"=w1101:u8, "Data[3]"=w1100:u8, "Data[4]"=w1099:u8, "Data[5]"=w1098:u8, "Data[6]"=w1097:u8)  [unwired: 1 out]
                n510 = To Word Integer(number=w1102) -> (16bit integer=w1115:i16)
                n511 = To Word Integer(number=w1098) -> (16bit integer=w1108:i16)
                n512 = To Word Integer(number=w1100) -> (16bit integer=w1111:i16)
                n513 = Rotate(1:w1115, 2:w1105) -> (0:w1114:i16)
                n514 = Rotate(1:w1108, 2:w1105) -> (0:w1107:i16)
                n515 = Rotate(1:w1111, 2:w1105) -> (0:w1110:i16)
                n516 = Add(x=w1114, y=w1101) -> (x+y=w1113:i16)
                n517 = Add(x=w1107, y=w1097) -> (x+y=w1106:i16)
                n518 = Add(x=w1110, y=w1099) -> (x+y=w1109:i16)
                n519 = Divide(x=w1113, y=w1104) -> (x/y=w1096:dbl)
                "A电流" <- w1096
                "A电流" <- w1096
                n520 = Divide(x=w1106, y=w1104) -> (x/y=w1094:dbl)
                "C电流" <- w1094
                "C电流" <- w1094
                n521 = Divide(x=w1109, y=w1104) -> (x/y=w1095:dbl)
                "B电流" <- w1095
                "B电流" <- w1095
                n522 = Build Array(w1096, w1095, w1094) -> (w1093:dbl[])
              }
              frame 51 {
                w1129 = i16 256
                w1128 = 8
                n523 = Array To Cluster(array=w1127) -> (cluster=w1136:T14)
                n524 = Unbundle By Name(w1136) -> ("Data[1]"=w1126:u8, "Data[2]"=w1125:u8, "Data[3]"=w1124:u8, "Data[4]"=w1123:u8, "Data[5]"=w1122:u8, "Data[6]"=w1121:u8)  [unwired: 1 out]
                n525 = To Unsigned Word Integer(number=w1126) -> (unsigned 16bit integer=w1139:u16)
                n526 = To Word Integer(number=w1124) -> (16bit integer=w1135:i16)
                n527 = To Word Integer(number=w1122) -> (16bit integer=w1132:i16)
                n528 = Rotate(1:w1139, 2:w1128) -> (0:w1138:u16)
                n529 = Rotate(1:w1135, 2:w1128) -> (0:w1134:i16)
                n530 = Rotate(1:w1132, 2:w1128) -> (0:w1131:i16)
                n531 = Add(x=w1138, y=w1125) -> (x+y=w1137:u16)
                n532 = Add(x=w1134, y=w1123) -> (x+y=w1133:i16)
                n533 = Add(x=w1131, y=w1121) -> (x+y=w1130:i16)
                n534 = Divide(x=w1137, y=i16 1024) -> (x/y=w1119:dbl)
                "供电电压" <- w1119
                n535 = Divide(x=w1133, y=w1129) -> (x/y=w1118:dbl)
                "Ialfa" <- w1118
                n536 = Divide(x=w1130, y=w1129) -> (x/y=w1117:dbl)
                "Ibeta" <- w1117
                n537 = Build Array(w1119, w1118, w1117) -> (w1116:dbl[])
              }
              frame 52 {
                w1143 = i16 256
                w1149 = 8
                n538 = Array To Cluster(array=w1144) -> (cluster=w1153:T14)
                n539 = Unbundle By Name(w1153) -> ("Data[1]"=w1148:u8, "Data[2]"=w1147:u8, "Data[3]"=w1146:u8, "Data[4]"=w1145:u8)  [unwired: 1 out]
                n540 = To Word Integer(number=w1148) -> (16bit integer=w1156:i16)
                n541 = To Word Integer(number=w1146) -> (16bit integer=w1152:i16)
                n542 = Rotate(1:w1156, 2:w1149) -> (0:w1155:i16)
                n543 = Rotate(1:w1152, 2:w1149) -> (0:w1151:i16)
                n544 = Add(x=w1155, y=w1147) -> (x+y=w1154:i16)
                n545 = Add(x=w1151, y=w1145) -> (x+y=w1150:i16)
                n546 = Divide(x=w1154, y=w1143) -> (x/y=w1141:dbl)
                "Iqnow" <- w1141
                n547 = Divide(x=w1150, y=w1143) -> (x/y=w1140:dbl)
                "Idnow" <- w1140
                n548 = Build Array(w1141, w1140) -> (w1142:dbl[])
              }
              frame 53 {
                w1166 = i16 1024
                w1165 = 8
                n549 = Array To Cluster(array=w1164) -> (cluster=w1170:T14)
                n550 = Unbundle By Name(w1170) -> ("Data[1]"=w1163:u8, "Data[2]"=w1162:u8, "Data[3]"=w1161:u8, "Data[4]"=w1160:u8)  [unwired: 1 out]
                n551 = To Word Integer(number=w1163) -> (16bit integer=w1173:i16)
                n552 = To Word Integer(number=w1161) -> (16bit integer=w1169:i16)
                n553 = Rotate(1:w1173, 2:w1165) -> (0:w1172:i16)
                n554 = Rotate(1:w1169, 2:w1165) -> (0:w1168:i16)
                n555 = Add(x=w1172, y=w1162) -> (x+y=w1171:i16)
                n556 = Add(x=w1168, y=w1160) -> (x+y=w1167:i16)
                n557 = Divide(x=w1171, y=w1166) -> (x/y=w1158:dbl)
                "Uq" <- w1158
                n558 = Divide(x=w1167, y=w1166) -> (x/y=w1157:dbl)
                "Ud" <- w1157
                n559 = Build Array(w1158, w1157) -> (w1159:dbl[])
              }
              frame 54 {
                w1183 = i16 1024
                w1182 = 8
                n560 = Array To Cluster(array=w1177) -> (cluster=w1187:T14)
                n561 = Unbundle By Name(w1187) -> ("Data[1]"=w1181:u8, "Data[2]"=w1180:u8, "Data[3]"=w1179:u8, "Data[4]"=w1178:u8)  [unwired: 1 out]
                n562 = To Word Integer(number=w1181) -> (16bit integer=w1190:i16)
                n563 = To Word Integer(number=w1179) -> (16bit integer=w1186:i16)
                n564 = Rotate(1:w1190, 2:w1182) -> (0:w1189:i16)
                n565 = Rotate(1:w1186, 2:w1182) -> (0:w1185:i16)
                n566 = Add(x=w1189, y=w1180) -> (x+y=w1188:i16)
                n567 = Add(x=w1185, y=w1178) -> (x+y=w1184:i16)
                n568 = Divide(x=w1188, y=w1183) -> (x/y=w1175:dbl)
                "Ualfa" <- w1175
                n569 = Divide(x=w1184, y=w1183) -> (x/y=w1174:dbl)
                "Ubate" <- w1174
                n570 = Build Array(w1175, w1174) -> (w1176:dbl[])
              }
              frame 55 {
                w1204 = u16 0
                w1203 = 8
                n571 = Array To Cluster(array=w1202) -> (cluster=w1211:T14)
                n572 = Unbundle By Name(w1211) -> ("Data[1]"=w1196:u8, "Data[2]"=w1197:u8, "Data[3]"=w1198:u8, "Data[4]"=w1199:u8, "Data[5]"=w1200:u8, "Data[6]"=w1201:u8, "Data[7]"=w1192:u8)  [unwired: 1 out]
                "sector" <- w1192
                n573 = To Word Integer(number=w1196) -> (16bit integer=w1214:i16)
                n574 = To Word Integer(number=w1198) -> (16bit integer=w1210:i16)
                n575 = To Word Integer(number=w1200) -> (16bit integer=w1207:i16)
                n576 = Rotate(1:w1214, 2:w1203) -> (0:w1213:i16)
                n577 = Rotate(1:w1210, 2:w1203) -> (0:w1209:i16)
                n578 = Rotate(1:w1207, 2:w1203) -> (0:w1206:i16)
                n579 = Add(x=w1213, y=w1197) -> (x+y=w1212:i16)
                n580 = Add(x=w1209, y=w1199) -> (x+y=w1208:i16)
                n581 = Add(x=w1206, y=w1201) -> (x+y=w1205:i16)
                n582 = Subtract ("减")(x=w1212, y=w1204) -> (x-y=w1195:u16)
                "PWM1" <- w1195
                n583 = Subtract ("减")(x=w1208, y=w1204) -> (x-y=w1194:u16)
                "PWM2" <- w1194
                n584 = Subtract ("减")(x=w1205, y=w1204) -> (x-y=w1193:u16)
                "PWM3" <- w1193
                n585 = Build Array(w1195, w1194, w1193, w1192) -> (w1191:u16[])
              }
              frame 56 {
                n586 = Array Subset(array=w1221, index=1, length=4) -> (w1218:u8[])
                n587 = Type Cast(type=2097152, x=w1218) -> (*(type *) &x=w1216:i32)
                "Sin" <- w1216
                "Cosin" <- w1216
                n588 = Build Array(w1216, w1216) -> (w1215:i32[])
              }
              frame 57 {
                n589 = Array To Cluster(array=w1238) -> (cluster=w1239:cluster{"Data[0]":u8, "Data[1]":u8})
                n590 = Unbundle By Name(w1239) -> ("Data[1]"=w1230:u8)  [unwired: 1 out]
                n591 = And(x=w1230, y=u8 56) -> (x .and. y?=w1233:u8)
                n592 = And(x=w1230, y=u8 192) -> (x .and. y?=w1236:u8)
                n593 = And(x=w1230, y=u8 7) -> (x .and. y?=w1227:u8)
                n594 = Logical Shift(y=i16 -3, x=w1233) -> (x << y=w1229:u8)
                n595 = Logical Shift(y=i16 -6, x=w1236) -> (x << y=w1225:u8)
                n596 = Divide(x=w1229, y=u8 10) -> (x/y=w1224:dbl)
                n597 = Divide(x=w1227, y=u8 100) -> (x/y=w1223:dbl)
                n598 = Compound Arithmetic op=ADD(w1225, w1224, w1223) -> (→"版本号":dbl)
              }
              frame 58 {
                n599 = Array To Cluster(array=w1242) -> (cluster=w1247:T14)
                n600 = Unbundle By Name(w1247) -> ("Data[1]"=w1245:u8, "Data[2]"=w1244:u8)  [unwired: 1 out]
                n601 = Join Numbers(hi=w1245, lo=w1244) -> ((hi.lo)=w1246:u16)
                n602 = To Unsigned Word Integer(number=w1246) -> (unsigned 16bit integer=w1243:u16)
                n603 = Multiply(x=w1243, y=0.0054931640625) -> (x*y=w1241:dbl)
                n604 = property on="机械角度" class="DigNum (严格)"("Value"=w1241) -> ()  [unwired: 2 in, 2 out]
              }
              frame 59 {
                n605 = Array To Cluster(array=w1249) -> (cluster=w1255:T14)
                n606 = Unbundle By Name(w1255) -> ("Data[1]"=w1253:u8, "Data[2]"=w1252:u8)  [unwired: 1 out]
                n607 = Join Numbers(hi=w1253, lo=w1252) -> ((hi.lo)=w1254:u16)
                n608 = To Word Integer(number=w1254) -> (16bit integer=w1251:i16)
                n609 = Divide(x=w1251, y=i16 1) -> (x/y=w1248:dbl)
                n610 = property on="转速" class="DigNum (严格)"("Value"=w1248) -> ()  [unwired: 2 in, 2 out]
              }
              frame 60 {
                n611 = Array To Cluster(array=w1257) -> (cluster=w1263:T14)
                n612 = Unbundle By Name(w1263) -> ("Data[1]"=w1261:u8, "Data[2]"=w1260:u8)  [unwired: 1 out]
                n613 = Join Numbers(hi=w1261, lo=w1260) -> ((hi.lo)=w1262:u16)
                n614 = To Word Integer(number=w1262) -> (16bit integer=w1259:i16)
                n615 = Divide(x=w1259, y=i16 256) -> (x/y=w1256:dbl)
                n616 = property on="Iqnow" class="DigNum (严格)"("Value"=w1256) -> ()  [unwired: 2 in, 2 out]
              }
              frame 61 {
                n617 = Array To Cluster(array=w1267) -> (cluster=w1271:T14)
                n618 = Unbundle By Name(w1271) -> ("Data[1]"=w1269:u8, "Data[2]"=w1268:u8)  [unwired: 1 out]
                n619 = Join Numbers(hi=w1269, lo=w1268) -> ((hi.lo)=w1270:u16)
                n620 = To Word Integer(number=w1270) -> (16bit integer=w1266:i16)
                n621 = Divide(x=w1266, y=i16 4) -> (x/y=→"温度":dbl)
              }
              frame 64 {
                n622 = Array To Cluster(array=w1273) -> (cluster=w1278:T14)
                n623 = Unbundle By Name(w1278) -> ("Data[1]"=w1274:u8, "Data[2]"=w1275:u8)  [unwired: 1 out]
                n624 = To Unsigned Word Integer(number=w1274) -> (unsigned 16bit integer=w1281:u16)
                n625 = Rotate(1:w1281, 2:8) -> (0:w1280:u16)
                n626 = Add ("加")(x=w1280, y=w1275) -> (x+y=w1279:u16)
                n627 = Divide(x=w1279, y=u16 256) -> (x/y=→"设定位置_回":dbl)
              }
              frame 65 {
                n628 = Array To Cluster(array=w1286) -> (cluster=w1287:T14)
                n629 = Unbundle By Name(w1287) -> ("Data[1]"=w1284:u8, "Data[2]"=w1283:u8)  [unwired: 1 out]
                n630 = Join Numbers(hi=w1284, lo=w1283) -> ((hi.lo)=w1285:u16)
                n631 = To Word Integer(number=w1285) -> (16bit integer=→"设定速度_回":i16)
              }
              frame 66 {
                n632 = Array To Cluster(array=w1289) -> (cluster=w1294:T14)
                n633 = Unbundle By Name(w1294) -> ("Data[1]"=w1290:u8, "Data[2]"=w1291:u8)  [unwired: 1 out]
                n634 = To Word Integer(number=w1290) -> (16bit integer=w1297:i16)
                n635 = Rotate(1:w1297, 2:8) -> (0:w1296:i16)
                n636 = Add ("加")(x=w1296, y=w1291) -> (x+y=w1295:i16)
                n637 = Divide(x=w1295, y=u16 256) -> (x/y=→"设定电流_回":dbl)
              }
              frame 81 {
                n638 = Array To Cluster(array=w1299) -> (cluster=w1304:T14)
                n639 = Unbundle By Name(w1304) -> ("Data[1]"=w1300:u8, "Data[2]"=w1301:u8)  [unwired: 1 out]
                n640 = To Unsigned Word Integer(number=w1300) -> (unsigned 16bit integer=w1307:u16)
                n641 = Rotate(1:w1307, 2:8) -> (0:w1306:u16)
                n642 = Add ("加")(x=w1306, y=w1301) -> (x+y=w1305:u16)
                n643 = Divide(x=w1305, y=u16 256) -> (x/y=→"电流环KP_回":dbl)
              }
              frame 82 {
                n644 = Array To Cluster(array=w1309) -> (cluster=w1314:T14)
                n645 = Unbundle By Name(w1314) -> ("Data[1]"=w1310:u8, "Data[2]"=w1311:u8)  [unwired: 1 out]
                n646 = To Unsigned Word Integer(number=w1310) -> (unsigned 16bit integer=w1317:u16)
                n647 = Rotate(1:w1317, 2:8) -> (0:w1316:u16)
                n648 = Add ("加")(x=w1316, y=w1311) -> (x+y=w1315:u16)
                n649 = Divide(x=w1315, y=u16 256) -> (x/y=→"电流环KI_回":dbl)
              }
              frame 83 {
                n650 = Array To Cluster(array=w1319) -> (cluster=w1324:T14)
                n651 = Unbundle By Name(w1324) -> ("Data[1]"=w1320:u8, "Data[2]"=w1321:u8)  [unwired: 1 out]
                n652 = To Unsigned Word Integer(number=w1320) -> (unsigned 16bit integer=w1327:u16)
                n653 = Rotate(1:w1327, 2:8) -> (0:w1326:u16)
                n654 = Add ("加")(x=w1326, y=w1321) -> (x+y=w1325:u16)
                n655 = Divide(x=w1325, y=u16 256) -> (x/y=→"速度环KP_回":dbl)
              }
              frame 84 {
                n656 = Array To Cluster(array=w1329) -> (cluster=w1334:T14)
                n657 = Unbundle By Name(w1334) -> ("Data[1]"=w1330:u8, "Data[2]"=w1331:u8)  [unwired: 1 out]
                n658 = To Unsigned Word Integer(number=w1330) -> (unsigned 16bit integer=w1337:u16)
                n659 = Rotate(1:w1337, 2:8) -> (0:w1336:u16)
                n660 = Add ("加")(x=w1336, y=w1331) -> (x+y=w1335:u16)
                n661 = Divide(x=w1335, y=u16 256) -> (x/y=→"速度环KI_回":dbl)
              }
              frame 85 {
                n662 = Array To Cluster(array=w1339) -> (cluster=w1344:T14)
                n663 = Unbundle By Name(w1344) -> ("Data[1]"=w1340:u8, "Data[2]"=w1341:u8)  [unwired: 1 out]
                n664 = To Unsigned Word Integer(number=w1340) -> (unsigned 16bit integer=w1347:u16)
                n665 = Rotate(1:w1347, 2:8) -> (0:w1346:u16)
                n666 = Add ("加")(x=w1346, y=w1341) -> (x+y=w1345:u16)
                n667 = Divide(x=w1345, y=u16 8) -> (x/y=→"加速度_回":dbl)
              }
              frame 90 {
                n668 = Array To Cluster(array=w1352) -> (cluster=w1353:T14)
                n669 = Unbundle By Name(w1353) -> ("Data[1]"=w1350:u8, "Data[2]"=w1349:u8)  [unwired: 1 out]
                n670 = Join Numbers(hi=w1350, lo=w1349) -> ((hi.lo)=w1351:u16)
                n671 = To Unsigned Word Integer(number=w1351) -> (unsigned 16bit integer=→"AI_K0_回":u16)
              }
              frame 91 {
                n672 = Array To Cluster(array=w1355) -> (cluster=w1359:T14)
                n673 = Unbundle By Name(w1359) -> ("Data[1]"=w1357:u8, "Data[2]"=w1356:u8)  [unwired: 1 out]
                n674 = Join Numbers(hi=w1357, lo=w1356) -> ((hi.lo)=w1358:u16)
                n675 = To Unsigned Word Integer(number=w1358) -> (unsigned 16bit integer=→"BI_K0_回":u16)
              }
              frame 92 {
                n676 = Array To Cluster(array=w1361) -> (cluster=w1365:T14)
                n677 = Unbundle By Name(w1365) -> ("Data[1]"=w1363:u8, "Data[2]"=w1362:u8)  [unwired: 1 out]
                n678 = Join Numbers(hi=w1363, lo=w1362) -> ((hi.lo)=w1364:u16)
                n679 = To Unsigned Word Integer(number=w1364) -> (unsigned 16bit integer=→"CI_K0_回":u16)
              }
            }
            n680 = case shown="真" w997 {
              tunnel: w996 -> [_ w1007]
              tunnel: w995 -> [_ w1005]
              frame False {
              }
              frame True {
                n681 = Array Size(array=w1005) -> (size(s)=w1006:i32)
                n682 = Open/Create/Replace File(file path (use dialog)=w1007, operation (0:open)=T11."open or create") -> (refnum out=w1015:refnum<file>, error out=w1004:errorcluster)  [unwired: 4 in, 1 out]
                n683 = for {
                  N: w1006 -> [_]
                  shift-right: [w1023] -> w1012
                  shift-left: "" -> [w1020]
                  tunnel: w1005 -> [w1018]
                  i -> [w1019]
                  # "浮点文本存储"
                  # "2-14"
                  n684 = Index Array(array=w1018, index=w1019) -> (element=w1017:dbl)
                  n685 = Number To Fractional String(number=w1017) -> (F-format string=w1022:string)  [unwired: 3 in]
                  n686 = Concatenate Strings(w1020, w1022, "\t") -> (w1023:string)
                }
                n687 = Set File Position(refnum=w1015, from (0:start)=u16 1, error in=w1004) -> (refnum out=w1014:refnum<file>, error out=w1003:errorcluster)  [unwired: 1 in]
                n688 = Concatenate Strings(w1012, "\r") -> (w1010:string)
                n689 = Write to Text File(file (use dialog)=w1014, text=w1010, error in=w1003) -> (refnum out=w1013:refnum<file>, error out=w1002:errorcluster)  [unwired: 1 in, 1 out]
                n690 = Close File(refnum=w1013, error in=w1002) -> (error out=w1001:errorcluster)  [unwired: 1 out]
                n691 = call <vilib>:"Clear Errors.vi"("error in (no error)"=w1001) -> ()  [unwired: 6 in, 1 out]
              }
            }
          }
        }
      }
      frame True {
      }
    }
  }
  n692 = while "接收线程" {
    tunnel: w9 -> [w1369]
    shift-right: [w1367] -> _
    shift-left: u32 0 ("RecvCnt") -> [w1368]
    stop <- "RcvEnable" continue-if-true
    n693 = local read "Open"() -> (w1370:bool)
    n694 = case shown="真" w1370 {
      tunnel: w1369 -> [_ w1377]
      tunnel: w1368 -> [w1372 w1376]
      tunnel: [w1372 w1375] -> w1367
      frame False {
        # "CAN未打开，延时50ms"
        n695 = Wait (ms)(milliseconds to wait=u32 50 ("等待时间（毫秒）")) -> ()  [unwired: 1 out]
      }
      frame True {
        n696 = local read "DevType"() -> (w1381:T5)
        n697 = local read "Channel"() -> (w1374:T4)
        n698 = call "VCI_Receive.vi"("CANIndex"=w1374, "DevIndex"=u32 0, "DevType"=w1381) -> ("Recieve"=w1378:T6[])  [unwired: 3 in, 5 out]
        n699 = Empty Array?(array=w1378) -> (empty?=w1379:bool)
        n700 = case shown="假" w1379 {
          tunnel: w1377 -> [w1388 _]
          tunnel: w1378 -> [w1383 _]
          tunnel: [w1387 _] -> _
          tunnel: w1376 -> [w1385 w1400]
          tunnel: [w1384 w1400] -> w1375
          tunnel: w1374 -> [w1386 _]
          frame False {
            n701 = Array Size(array=w1383) -> (size(s)=w1382:i32)
            n702 = for {
              N: w1382 -> [_]
              tunnel: w1388 -> [w1399]
              tunnel: [w1397] -> w1387 mode=indexing
              tunnel: w1383 -> [w1392]
              tunnel: w1386 -> [w1396]
              shift-right: [w1393] -> w1384
              shift-left: w1385 -> [w1394]
              i -> [w1390]
              n703 = Array Subset(array=w1392, index=w1390, length=1) -> (w1391:T6[])
              n704 = Increment(x=w1394) -> (x+1=w1393:u32)
              n705 = call "Demo_MakeDispBuff.vi"("Channel"=w1396, "Type"=enum16{"接收", "发送"}."接收", "OBJs"=w1391) -> ("Buffer"=w1398:T7)
              n706 = Enqueue Element(queue=w1399, element=w1398) -> (error out=w1397:errorcluster)  [unwired: 1 in, 3 out]
            }
            "RecvCnt" <- w1384
          }
          frame True {
          }
        }
      }
    }
  }
  n707 = control-ref of="本应用程序"() -> (w6:refnum<vi>)
  n708 = invoke class="VI" method="FP.Close"(error in=w4) -> (error out=w3:errorcluster)  [unwired: 2 in, 2 out]
  n709 = property class="App"(reference=w6) -> ("App.Kind"=w5:T16)  [unwired: 1 in, 2 out]
  n710 = case shown="\"Development System\"" w5 {
    tunnel: w3 -> [_ _]
    frame "invalid app kind", Default {
      n711 = Quit LabVIEW() -> ()  [unwired: 1 out]
    }
    frame "Development System" {
    }
  }
